vi "Sparameter Testing.vi"(0 "VNA Model:":enum16{"E5071C", "N5230A(C)", "N5224A"}(ring)=enum."N5224A", 1 "VNA VISA":refnum<visa-resource-name>="TCPIP0::A-N5224A-41544.local::hislip0::INSTR", 2 "Port Type":u16(ring), 3 "Reference":T2, 4 "VISA COM":refnum<visa-resource-name>="COM3", 5 "Channel":string="1", 6 "Information In":T1={"Sample PN: "="", "SampleSN:"="", "Sparam Test Item"=[], "S-para Pair Name"=[], "Length"="", "Diff Test Item Name"=["SDD21", "SDD22", "SCD21", "SCD22", "SCC11", "NEXT", "FEXT"], "Diff Test Item Name smooth"=[], "smooth point"=0.0, "limitSpec"=[], "switchIndexOffset"=0, "testType"=enum."Loss", "pairStartIndex"=0, "DAQ  Model:"=enum."NI PCI-6509", "VISA COM"="COM3", "Matrix  In"=[]}, 7 "TDR setting array":T3(array[cluster]), 8 "Mode(Demo,Manual)":T7, 9 "DAQ  Model:":T6(ring), 10 "S4P Data Type":enum16{"THRU", "NEXT", "FEXT"}(ring), 11 "Matrix  In":T8, 12 "ILDSpec":enum16{"IEEE802.3ba", "FDR", "EDR"}(ring), 13 "Option":T5, 14 "MulChannel?":bool, 15 "2X Thru":dbl[](array[numeric]), 16 "proBar_ref":refnum<vi>) -> (17 "String data":string, 18 "Basic Path":path, 19 "S4P_TXT_ Data":string[](array[string]), 20 "Frequency(Hz)":dbl[](array[numeric]), 21 "Data Out":dbl[][][](array[numeric]), 22 "Testing Results":bool[](array[boolean]), 24 "Total Reult":bool, 25 "TXT Data Path":path, 26 "Items Result":string[](array[string]), 27 "S4P Data Path":path)   [LabVIEW 2011]
uses:
  dataType/informationIn.ctl
  <userlib>/_OpenG.lib/array/array.llb/Delete Elements from 2D Array (DBL)__ogtk.vi
  <vilib>/Utility/file.llb/Write To Spreadsheet File (DBL).vi
  <vilib>/Utility/file.llb/Write To Spreadsheet File (string).vi
panel:
  in  "delay array":dbl[](array[numeric])
  out "Time Array 4":dbl[](array[numeric])
  out "Time Array 3":dbl[](array[numeric])
  out "NextSourced":dbl[][](array[numeric])
  in  "NEXT source":dbl[][](array[numeric])
  out "smoothed Diff Data":dbl[](array[numeric])
  out "ILD_15 graph index":i32
  out "reslut_TDD22toTDD11 2":bool
  out "reslut_TDD11toTDD22":bool
  out "1d reslut":bool[](array[boolean])
  out "TDD22toTDD11":dbl[](array[numeric])
  out "TDD11toTDD22":dbl[](array[numeric])
  out "Dataout":dbl[][](array[numeric])
  out "sparaLength":dbl
  in  "TDR Setting 2":T4
  out "Time Array 2":dbl[](array[numeric])
  out "SDD21 For ILD_15":dbl[][](array[numeric])
  out "大小":i32
  out "ILD_15%":bool[](array[boolean])
  out "ILD":dbl[][](array[numeric])
  out "Graph Size":i32
  in  "Skew result":dbl[](array[numeric])
  out "Skew Time":dbl[](array[numeric])=[4.0, 4.0015003751, 4.0030007502, 4.0045011253, 4.0060015004, 4.0075018755, 4.0090022506, 4.0105026257, 4.0120030008, 4.0135033758, 4.0150037509, 4.016504126, 4.0180045011, 4.0195048762, 4.0210052513, 4.0225056264, 4.0240060015, 4.0255063766, 4.0270067517, 4.0285071268, 4.0300075019, 4.031507877, 4.0330082521, 4.0345086272, 4.0360090023, 4.0375093773, 4.0390097524, 4.0405101275, 4.0420105026, 4.0435108777, 4.0450112528, 4.0465116279, 4.048012003, 4.0495123781, 4.0510127532, 4.0525131283, 4.0540135034, 4.0555138785, 4.0570142536, 4.0585146287, 4.0600150038, 4.0615153788, 4.0630157539, 4.064516129, 4.0660165041, 4.0675168792, 4.0690172543, 4.0705176294, 4.0720180045, 4.0735183796, 4.0750187547, 4.0765191298, 4.0780195049, 4.07951988, 4.0810202551, 4.0825206302, 4.0840210053, 4.0855213803, 4.0870217554, 4.0885221305, 4.0900225056, 4.0915228807, 4.0930232558, 4.0945236309, 4.096024006, 4.0975243811, 4.0990247562, 4.1005251313, 4.1020255064, 4.1035258815, 4.1050262566, 4.1065266317, 4.1080270068, 4.1095273818, 4.1110277569, 4.112528132, 4.1140285071, 4.1155288822, 4.1170292573, 4.1185296324, 4.1200300075, 4.1215303826, 4.1230307577, 4.1245311328, 4.1260315079, 4.127531883, 4.1290322581, 4.1305326332, 4.1320330083, 4.1335333833, 4.1350337584, 4.1365341335, 4.1380345086, 4.1395348837, 4.1410352588, 4.1425356339, 4.144036009, 4.1455363841, 4.1470367592, 4.1485371343, 4.1500375094, 4.1515378845, 4.1530382596, 4.1545386347, 4.1560390098, 4.1575393848, 4.1590397599, 4.160540135, 4.1620405101, 4.1635408852, 4.1650412603, 4.1665416354, 4.1680420105, 4.1695423856, 4.1710427607, 4.1725431358, 4.1740435109, 4.175543886, 4.1770442611, 4.1785446362, 4.1800450113, 4.1815453863, 4.1830457614, 4.1845461365, 4.1860465116, 4.1875468867, 4.1890472618, 4.1905476369, 4.192048012, 4.1935483871, 4.1950487622, 4.1965491373, 4.1980495124, 4.1995498875, 4.2010502626, 4.2025506377, 4.2040510128, 4.2055513878, 4.2070517629, 4.208552138, 4.2100525131, 4.2115528882, 4.2130532633, 4.2145536384, 4.2160540135, 4.2175543886, 4.2190547637, 4.2205551388, 4.2220555139, 4.223555889, 4.2250562641, 4.2265566392, 4.2280570143, 4.2295573893, 4.2310577644, 4.2325581395, 4.2340585146, 4.2355588897, 4.2370592648, 4.2385596399, 4.240060015, 4.2415603901, 4.2430607652, 4.2445611403, 4.2460615154, 4.2475618905, 4.2490622656, 4.2505626407, 4.2520630158, 4.2535633908, 4.2550637659, 4.256564141, 4.2580645161, 4.2595648912, 4.2610652663, 4.2625656414, 4.2640660165, 4.2655663916, 4.2670667667, 4.2685671418, 4.2700675169, 4.271567892, 4.2730682671, 4.2745686422, 4.2760690173, 4.2775693923, 4.2790697674, 4.2805701425, 4.2820705176, 4.2835708927, 4.2850712678, 4.2865716429, 4.288072018, 4.2895723931, 4.2910727682, 4.2925731433, 4.2940735184, 4.2955738935, 4.2970742686, 4.2985746437, 4.3000750188, 4.3015753938, 4.3030757689, 4.304576144, 4.3060765191, 4.3075768942, 4.3090772693, 4.3105776444, 4.3120780195, 4.3135783946, 4.3150787697, 4.3165791448, 4.3180795199, 4.319579895, 4.3210802701, 4.3225806452, 4.3240810203, 4.3255813953, 4.3270817704, 4.3285821455, 4.3300825206, 4.3315828957, 4.3330832708, 4.3345836459, 4.336084021, 4.3375843961, 4.3390847712, 4.3405851463, 4.3420855214, 4.3435858965, 4.3450862716, 4.3465866467, 4.3480870218, 4.3495873968, 4.3510877719, 4.352588147, 4.3540885221, 4.3555888972, 4.3570892723, 4.3585896474, 4.3600900225, 4.3615903976, 4.3630907727, 4.3645911478, 4.3660915229, 4.367591898, 4.3690922731, 4.3705926482, 4.3720930233, 4.3735933983, 4.3750937734, 4.3765941485, 4.3780945236, 4.3795948987, 4.3810952738, 4.3825956489, 4.384096024, 4.3855963991, 4.3870967742, 4.3885971493, 4.3900975244, 4.3915978995, 4.3930982746, 4.3945986497, 4.3960990248, 4.3975993998, 4.3990997749, 4.40060015, 4.4021005251, 4.4036009002, 4.4051012753, 4.4066016504, 4.4081020255, 4.4096024006, 4.4111027757, 4.4126031508, 4.4141035259, 4.415603901, 4.4171042761, 4.4186046512, 4.4201050263, 4.4216054014, 4.4231057764, 4.4246061515, 4.4261065266, 4.4276069017, 4.4291072768, 4.4306076519, 4.432108027, 4.4336084021, 4.4351087772, 4.4366091523, 4.4381095274, 4.4396099025, 4.4411102776, 4.4426106527, 4.4441110278, 4.4456114029, 4.4471117779, 4.448612153, 4.4501125281, 4.4516129032, 4.4531132783, 4.4546136534, 4.4561140285, 4.4576144036, 4.4591147787, 4.4606151538, 4.4621155289, 4.463615904, 4.4651162791, 4.4666166542, 4.4681170293, 4.4696174044, 4.4711177794, 4.4726181545, 4.4741185296, 4.4756189047, 4.4771192798, 4.4786196549, 4.48012003, 4.4816204051, 4.4831207802, 4.4846211553, 4.4861215304, 4.4876219055, 4.4891222806, 4.4906226557, 4.4921230308, 4.4936234059, 4.4951237809, 4.496624156, 4.4981245311, 4.4996249062, 4.5011252813, 4.5026256564, 4.5041260315, 4.5056264066, 4.5071267817, 4.5086271568, 4.5101275319, 4.511627907, 4.5131282821, 4.5146286572, 4.5161290323, 4.5176294074, 4.5191297824, 4.5206301575, 4.5221305326, 4.5236309077, 4.5251312828, 4.5266316579, 4.528132033, 4.5296324081, 4.5311327832, 4.5326331583, 4.5341335334, 4.5356339085, 4.5371342836, 4.5386346587, 4.5401350338, 4.5416354089, 4.5431357839, 4.544636159, 4.5461365341, 4.5476369092, 4.5491372843, 4.5506376594, 4.5521380345, 4.5536384096, 4.5551387847, 4.5566391598, 4.5581395349, 4.55963991, 4.5611402851, 4.5626406602, 4.5641410353, 4.5656414104, 4.5671417854, 4.5686421605, 4.5701425356, 4.5716429107, 4.5731432858, 4.5746436609, 4.576144036, 4.5776444111, 4.5791447862, 4.5806451613, 4.5821455364, 4.5836459115, 4.5851462866, 4.5866466617, 4.5881470368, 4.5896474119, 4.5911477869, 4.592648162, 4.5941485371, 4.5956489122, 4.5971492873, 4.5986496624, 4.6001500375, 4.6016504126, 4.6031507877, 4.6046511628, 4.6061515379, 4.607651913, 4.6091522881, 4.6106526632, 4.6121530383, 4.6136534134, 4.6151537884, 4.6166541635, 4.6181545386, 4.6196549137, 4.6211552888, 4.6226556639, 4.624156039, 4.6256564141, 4.6271567892, 4.6286571643, 4.6301575394, 4.6316579145, 4.6331582896, 4.6346586647, 4.6361590398, 4.6376594149, 4.6391597899, 4.640660165, 4.6421605401, 4.6436609152, 4.6451612903, 4.6466616654, 4.6481620405, 4.6496624156, 4.6511627907, 4.6526631658, 4.6541635409, 4.655663916, 4.6571642911, 4.6586646662, 4.6601650413, 4.6616654164, 4.6631657914, 4.6646661665, 4.6661665416, 4.6676669167, 4.6691672918, 4.6706676669, 4.672168042, 4.6736684171, 4.6751687922, 4.6766691673, 4.6781695424, 4.6796699175, 4.6811702926, 4.6826706677, 4.6841710428, 4.6856714179, 4.6871717929, 4.688672168, 4.6901725431, 4.6916729182, 4.6931732933, 4.6946736684, 4.6961740435, 4.6976744186, 4.6991747937, 4.7006751688, 4.7021755439, 4.703675919, 4.7051762941, 4.7066766692, 4.7081770443, 4.7096774194, 4.7111777944, 4.7126781695, 4.7141785446, 4.7156789197, 4.7171792948, 4.7186796699, 4.720180045, 4.7216804201, 4.7231807952, 4.7246811703, 4.7261815454, 4.7276819205, 4.7291822956, 4.7306826707, 4.7321830458, 4.7336834209, 4.7351837959, 4.736684171, 4.7381845461, 4.7396849212, 4.7411852963, 4.7426856714, 4.7441860465, 4.7456864216, 4.7471867967, 4.7486871718, 4.7501875469, 4.751687922, 4.7531882971, 4.7546886722, 4.7561890473, 4.7576894224, 4.7591897974, 4.7606901725, 4.7621905476, 4.7636909227, 4.7651912978, 4.7666916729, 4.768192048, 4.7696924231, 4.7711927982, 4.7726931733, 4.7741935484, 4.7756939235, 4.7771942986, 4.7786946737, 4.7801950488, 4.7816954239, 4.7831957989, 4.784696174, 4.7861965491, 4.7876969242, 4.7891972993, 4.7906976744, 4.7921980495, 4.7936984246, 4.7951987997, 4.7966991748, 4.7981995499, 4.799699925, 4.8012003001, 4.8027006752, 4.8042010503, 4.8057014254, 4.8072018005, 4.8087021755, 4.8102025506, 4.8117029257, 4.8132033008, 4.8147036759, 4.816204051, 4.8177044261, 4.8192048012, 4.8207051763, 4.8222055514, 4.8237059265, 4.8252063016, 4.8267066767, 4.8282070518, 4.8297074269, 4.831207802, 4.832708177, 4.8342085521, 4.8357089272, 4.8372093023, 4.8387096774, 4.8402100525, 4.8417104276, 4.8432108027, 4.8447111778, 4.8462115529, 4.847711928, 4.8492123031, 4.8507126782, 4.8522130533, 4.8537134284, 4.8552138035, 4.8567141785, 4.8582145536, 4.8597149287, 4.8612153038, 4.8627156789, 4.864216054, 4.8657164291, 4.8672168042, 4.8687171793, 4.8702175544, 4.8717179295, 4.8732183046, 4.8747186797, 4.8762190548, 4.8777194299, 4.879219805, 4.88072018, 4.8822205551, 4.8837209302, 4.8852213053, 4.8867216804, 4.8882220555, 4.8897224306, 4.8912228057, 4.8927231808, 4.8942235559, 4.895723931, 4.8972243061, 4.8987246812, 4.9002250563, 4.9017254314, 4.9032258065, 4.9047261815, 4.9062265566, 4.9077269317, 4.9092273068, 4.9107276819, 4.912228057, 4.9137284321, 4.9152288072, 4.9167291823, 4.9182295574, 4.9197299325, 4.9212303076, 4.9227306827, 4.9242310578, 4.9257314329, 4.927231808, 4.928732183, 4.9302325581, 4.9317329332, 4.9332333083, 4.9347336834, 4.9362340585, 4.9377344336, 4.9392348087, 4.9407351838, 4.9422355589, 4.943735934, 4.9452363091, 4.9467366842, 4.9482370593, 4.9497374344, 4.9512378095, 4.9527381845, 4.9542385596, 4.9557389347, 4.9572393098, 4.9587396849, 4.96024006, 4.9617404351, 4.9632408102, 4.9647411853, 4.9662415604, 4.9677419355, 4.9692423106, 4.9707426857, 4.9722430608, 4.9737434359, 4.975243811, 4.976744186, 4.9782445611, 4.9797449362, 4.9812453113, 4.9827456864, 4.9842460615, 4.9857464366, 4.9872468117, 4.9887471868, 4.9902475619, 4.991747937, 4.9932483121, 4.9947486872, 4.9962490623, 4.9977494374, 4.9992498125, 5.0007501875, 5.0022505626, 5.0037509377, 5.0052513128, 5.0067516879, 5.008252063, 5.0097524381, 5.0112528132, 5.0127531883, 5.0142535634, 5.0157539385, 5.0172543136, 5.0187546887, 5.0202550638, 5.0217554389, 5.023255814, 5.024756189, 5.0262565641, 5.0277569392, 5.0292573143, 5.0307576894, 5.0322580645, 5.0337584396, 5.0352588147, 5.0367591898, 5.0382595649, 5.03975994, 5.0412603151, 5.0427606902, 5.0442610653, 5.0457614404, 5.0472618155, 5.0487621905, 5.0502625656, 5.0517629407, 5.0532633158, 5.0547636909, 5.056264066, 5.0577644411, 5.0592648162, 5.0607651913, 5.0622655664, 5.0637659415, 5.0652663166, 5.0667666917, 5.0682670668, 5.0697674419, 5.071267817, 5.072768192, 5.0742685671, 5.0757689422, 5.0772693173, 5.0787696924, 5.0802700675, 5.0817704426, 5.0832708177, 5.0847711928, 5.0862715679, 5.087771943, 5.0892723181, 5.0907726932, 5.0922730683, 5.0937734434, 5.0952738185, 5.0967741935, 5.0982745686, 5.0997749437, 5.1012753188, 5.1027756939, 5.104276069, 5.1057764441, 5.1072768192, 5.1087771943, 5.1102775694, 5.1117779445, 5.1132783196, 5.1147786947, 5.1162790698, 5.1177794449, 5.11927982, 5.120780195, 5.1222805701, 5.1237809452, 5.1252813203, 5.1267816954, 5.1282820705, 5.1297824456, 5.1312828207, 5.1327831958, 5.1342835709, 5.135783946, 5.1372843211, 5.1387846962, 5.1402850713, 5.1417854464, 5.1432858215, 5.1447861965, 5.1462865716, 5.1477869467, 5.1492873218, 5.1507876969, 5.152288072, 5.1537884471, 5.1552888222, 5.1567891973, 5.1582895724, 5.1597899475, 5.1612903226, 5.1627906977, 5.1642910728, 5.1657914479, 5.167291823, 5.168792198, 5.1702925731, 5.1717929482, 5.1732933233, 5.1747936984, 5.1762940735, 5.1777944486, 5.1792948237, 5.1807951988, 5.1822955739, 5.183795949, 5.1852963241, 5.1867966992, 5.1882970743, 5.1897974494, 5.1912978245, 5.1927981995, 5.1942985746, 5.1957989497, 5.1972993248, 5.1987996999, 5.200300075, 5.2018004501, 5.2033008252, 5.2048012003, 5.2063015754, 5.2078019505, 5.2093023256, 5.2108027007, 5.2123030758, 5.2138034509, 5.215303826, 5.2168042011, 5.2183045761, 5.2198049512, 5.2213053263, 5.2228057014, 5.2243060765, 5.2258064516, 5.2273068267, 5.2288072018, 5.2303075769, 5.231807952, 5.2333083271, 5.2348087022, 5.2363090773, 5.2378094524, 5.2393098275, 5.2408102026, 5.2423105776, 5.2438109527, 5.2453113278, 5.2468117029, 5.248312078, 5.2498124531, 5.2513128282, 5.2528132033, 5.2543135784, 5.2558139535, 5.2573143286, 5.2588147037, 5.2603150788, 5.2618154539, 5.263315829, 5.2648162041, 5.2663165791, 5.2678169542, 5.2693173293, 5.2708177044, 5.2723180795, 5.2738184546, 5.2753188297, 5.2768192048, 5.2783195799, 5.279819955, 5.2813203301, 5.2828207052, 5.2843210803, 5.2858214554, 5.2873218305, 5.2888222056, 5.2903225806, 5.2918229557, 5.2933233308, 5.2948237059, 5.296324081, 5.2978244561, 5.2993248312, 5.3008252063, 5.3023255814, 5.3038259565, 5.3053263316, 5.3068267067, 5.3083270818, 5.3098274569, 5.311327832, 5.3128282071, 5.3143285821, 5.3158289572, 5.3173293323, 5.3188297074, 5.3203300825, 5.3218304576, 5.3233308327, 5.3248312078, 5.3263315829, 5.327831958, 5.3293323331, 5.3308327082, 5.3323330833, 5.3338334584, 5.3353338335, 5.3368342086, 5.3383345836, 5.3398349587, 5.3413353338, 5.3428357089, 5.344336084, 5.3458364591, 5.3473368342, 5.3488372093, 5.3503375844, 5.3518379595, 5.3533383346, 5.3548387097, 5.3563390848, 5.3578394599, 5.359339835, 5.3608402101, 5.3623405851, 5.3638409602, 5.3653413353, 5.3668417104, 5.3683420855, 5.3698424606, 5.3713428357, 5.3728432108, 5.3743435859, 5.375843961, 5.3773443361, 5.3788447112, 5.3803450863, 5.3818454614, 5.3833458365, 5.3848462116, 5.3863465866, 5.3878469617, 5.3893473368, 5.3908477119, 5.392348087, 5.3938484621, 5.3953488372, 5.3968492123, 5.3983495874, 5.3998499625, 5.4013503376, 5.4028507127, 5.4043510878, 5.4058514629, 5.407351838, 5.4088522131, 5.4103525881, 5.4118529632, 5.4133533383, 5.4148537134, 5.4163540885, 5.4178544636, 5.4193548387, 5.4208552138, 5.4223555889, 5.423855964, 5.4253563391, 5.4268567142, 5.4283570893, 5.4298574644, 5.4313578395, 5.4328582146, 5.4343585896, 5.4358589647, 5.4373593398, 5.4388597149, 5.44036009, 5.4418604651, 5.4433608402, 5.4448612153, 5.4463615904, 5.4478619655, 5.4493623406, 5.4508627157, 5.4523630908, 5.4538634659, 5.455363841, 5.4568642161, 5.4583645911, 5.4598649662, 5.4613653413, 5.4628657164, 5.4643660915, 5.4658664666, 5.4673668417, 5.4688672168, 5.4703675919, 5.471867967, 5.4733683421, 5.4748687172, 5.4763690923, 5.4778694674, 5.4793698425, 5.4808702176, 5.4823705926, 5.4838709677, 5.4853713428, 5.4868717179, 5.488372093, 5.4898724681, 5.4913728432, 5.4928732183, 5.4943735934, 5.4958739685, 5.4973743436, 5.4988747187, 5.5003750938, 5.5018754689, 5.503375844, 5.5048762191, 5.5063765941, 5.5078769692, 5.5093773443, 5.5108777194, 5.5123780945, 5.5138784696, 5.5153788447, 5.5168792198, 5.5183795949, 5.51987997, 5.5213803451, 5.5228807202, 5.5243810953, 5.5258814704, 5.5273818455, 5.5288822206, 5.5303825956, 5.5318829707, 5.5333833458, 5.5348837209, 5.536384096, 5.5378844711, 5.5393848462, 5.5408852213, 5.5423855964, 5.5438859715, 5.5453863466, 5.5468867217, 5.5483870968, 5.5498874719, 5.551387847, 5.5528882221, 5.5543885971, 5.5558889722, 5.5573893473, 5.5588897224, 5.5603900975, 5.5618904726, 5.5633908477, 5.5648912228, 5.5663915979, 5.567891973, 5.5693923481, 5.5708927232, 5.5723930983, 5.5738934734, 5.5753938485, 5.5768942236, 5.5783945986, 5.5798949737, 5.5813953488, 5.5828957239, 5.584396099, 5.5858964741, 5.5873968492, 5.5888972243, 5.5903975994, 5.5918979745, 5.5933983496, 5.5948987247, 5.5963990998, 5.5978994749, 5.59939985, 5.6009002251, 5.6024006002, 5.6039009752, 5.6054013503, 5.6069017254, 5.6084021005, 5.6099024756, 5.6114028507, 5.6129032258, 5.6144036009, 5.615903976, 5.6174043511, 5.6189047262, 5.6204051013, 5.6219054764, 5.6234058515, 5.6249062266, 5.6264066017, 5.6279069767, 5.6294073518, 5.6309077269, 5.632408102, 5.6339084771, 5.6354088522, 5.6369092273, 5.6384096024, 5.6399099775, 5.6414103526, 5.6429107277, 5.6444111028, 5.6459114779, 5.647411853, 5.6489122281, 5.6504126032, 5.6519129782, 5.6534133533, 5.6549137284, 5.6564141035, 5.6579144786, 5.6594148537, 5.6609152288, 5.6624156039, 5.663915979, 5.6654163541, 5.6669167292, 5.6684171043, 5.6699174794, 5.6714178545, 5.6729182296, 5.6744186047, 5.6759189797, 5.6774193548, 5.6789197299, 5.680420105, 5.6819204801, 5.6834208552, 5.6849212303, 5.6864216054, 5.6879219805, 5.6894223556, 5.6909227307, 5.6924231058, 5.6939234809, 5.695423856, 5.6969242311, 5.6984246062, 5.6999249812, 5.7014253563, 5.7029257314, 5.7044261065, 5.7059264816, 5.7074268567, 5.7089272318, 5.7104276069, 5.711927982, 5.7134283571, 5.7149287322, 5.7164291073, 5.7179294824, 5.7194298575, 5.7209302326, 5.7224306077, 5.7239309827, 5.7254313578, 5.7269317329, 5.728432108, 5.7299324831, 5.7314328582, 5.7329332333, 5.7344336084, 5.7359339835, 5.7374343586, 5.7389347337, 5.7404351088, 5.7419354839, 5.743435859, 5.7449362341, 5.7464366092, 5.7479369842, 5.7494373593, 5.7509377344, 5.7524381095, 5.7539384846, 5.7554388597, 5.7569392348, 5.7584396099, 5.759939985, 5.7614403601, 5.7629407352, 5.7644411103, 5.7659414854, 5.7674418605, 5.7689422356, 5.7704426107, 5.7719429857, 5.7734433608, 5.7749437359, 5.776444111, 5.7779444861, 5.7794448612, 5.7809452363, 5.7824456114, 5.7839459865, 5.7854463616, 5.7869467367, 5.7884471118, 5.7899474869, 5.791447862, 5.7929482371, 5.7944486122, 5.7959489872, 5.7974493623, 5.7989497374, 5.8004501125, 5.8019504876, 5.8034508627, 5.8049512378, 5.8064516129, 5.807951988, 5.8094523631, 5.8109527382, 5.8124531133, 5.8139534884, 5.8154538635, 5.8169542386, 5.8184546137, 5.8199549887, 5.8214553638, 5.8229557389, 5.824456114, 5.8259564891, 5.8274568642, 5.8289572393, 5.8304576144, 5.8319579895, 5.8334583646, 5.8349587397, 5.8364591148, 5.8379594899, 5.839459865, 5.8409602401, 5.8424606152, 5.8439609902, 5.8454613653, 5.8469617404, 5.8484621155, 5.8499624906, 5.8514628657, 5.8529632408, 5.8544636159, 5.855963991, 5.8574643661, 5.8589647412, 5.8604651163, 5.8619654914, 5.8634658665, 5.8649662416, 5.8664666167, 5.8679669917, 5.8694673668, 5.8709677419, 5.872468117, 5.8739684921, 5.8754688672, 5.8769692423, 5.8784696174, 5.8799699925, 5.8814703676, 5.8829707427, 5.8844711178, 5.8859714929, 5.887471868, 5.8889722431, 5.8904726182, 5.8919729932, 5.8934733683, 5.8949737434, 5.8964741185, 5.8979744936, 5.8994748687, 5.9009752438, 5.9024756189, 5.903975994, 5.9054763691, 5.9069767442, 5.9084771193, 5.9099774944, 5.9114778695, 5.9129782446, 5.9144786197, 5.9159789947, 5.9174793698, 5.9189797449, 5.92048012, 5.9219804951, 5.9234808702, 5.9249812453, 5.9264816204, 5.9279819955, 5.9294823706, 5.9309827457, 5.9324831208, 5.9339834959, 5.935483871, 5.9369842461, 5.9384846212, 5.9399849962, 5.9414853713, 5.9429857464, 5.9444861215, 5.9459864966, 5.9474868717, 5.9489872468, 5.9504876219, 5.951987997, 5.9534883721, 5.9549887472, 5.9564891223, 5.9579894974, 5.9594898725, 5.9609902476, 5.9624906227, 5.9639909977, 5.9654913728, 5.9669917479, 5.968492123, 5.9699924981, 5.9714928732, 5.9729932483, 5.9744936234, 5.9759939985, 5.9774943736, 5.9789947487, 5.9804951238, 5.9819954989, 5.983495874, 5.9849962491, 5.9864966242, 5.9879969992, 5.9894973743, 5.9909977494, 5.9924981245, 5.9939984996, 5.9954988747, 5.9969992498, 5.9984996249, 6.0, 6.0015003751, 6.0030007502, 6.0045011253, 6.0060015004, 6.0075018755, 6.0090022506, 6.0105026257, 6.0120030008, 6.0135033758, 6.0150037509, 6.016504126, 6.0180045011, 6.0195048762, 6.0210052513, 6.0225056264, 6.0240060015, 6.0255063766, 6.0270067517, 6.0285071268, 6.0300075019, 6.031507877, 6.0330082521, 6.0345086272, 6.0360090023, 6.0375093773, 6.0390097524, 6.0405101275, 6.0420105026, 6.0435108777, 6.0450112528, 6.0465116279, 6.048012003, 6.0495123781, 6.0510127532, 6.0525131283, 6.0540135034, 6.0555138785, 6.0570142536, 6.0585146287, 6.0600150038, 6.0615153788, 6.0630157539, 6.064516129, 6.0660165041, 6.0675168792, 6.0690172543, 6.0705176294, 6.0720180045, 6.0735183796, 6.0750187547, 6.0765191298, 6.0780195049, 6.07951988, 6.0810202551, 6.0825206302, 6.0840210053, 6.0855213803, 6.0870217554, 6.0885221305, 6.0900225056, 6.0915228807, 6.0930232558, 6.0945236309, 6.096024006, 6.0975243811, 6.0990247562, 6.1005251313, 6.1020255064, 6.1035258815, 6.1050262566, 6.1065266317, 6.1080270068, 6.1095273818, 6.1110277569, 6.112528132, 6.1140285071, 6.1155288822, 6.1170292573, 6.1185296324, 6.1200300075, 6.1215303826, 6.1230307577, 6.1245311328, 6.1260315079, 6.127531883, 6.1290322581, 6.1305326332, 6.1320330083, 6.1335333833, 6.1350337584, 6.1365341335, 6.1380345086, 6.1395348837, 6.1410352588, 6.1425356339, 6.144036009, 6.1455363841, 6.1470367592, 6.1485371343, 6.1500375094, 6.1515378845, 6.1530382596, 6.1545386347, 6.1560390098, 6.1575393848, 6.1590397599, 6.160540135, 6.1620405101, 6.1635408852, 6.1650412603, 6.1665416354, 6.1680420105, 6.1695423856, 6.1710427607, 6.1725431358, 6.1740435109, 6.175543886, 6.1770442611, 6.1785446362, 6.1800450113, 6.1815453863, 6.1830457614, 6.1845461365, 6.1860465116, 6.1875468867, 6.1890472618, 6.1905476369, 6.192048012, 6.1935483871, 6.1950487622, 6.1965491373, 6.1980495124, 6.1995498875, 6.2010502626, 6.2025506377, 6.2040510128, 6.2055513878, 6.2070517629, 6.208552138, 6.2100525131, 6.2115528882, 6.2130532633, 6.2145536384, 6.2160540135, 6.2175543886, 6.2190547637, 6.2205551388, 6.2220555139, 6.223555889, 6.2250562641, 6.2265566392, 6.2280570143, 6.2295573893, 6.2310577644, 6.2325581395, 6.2340585146, 6.2355588897, 6.2370592648, 6.2385596399, 6.240060015, 6.2415603901, 6.2430607652, 6.2445611403, 6.2460615154, 6.2475618905, 6.2490622656, 6.2505626407, 6.2520630158, 6.2535633908, 6.2550637659, 6.256564141, 6.2580645161, 6.2595648912, 6.2610652663, 6.2625656414, 6.2640660165, 6.2655663916, 6.2670667667, 6.2685671418, 6.2700675169, 6.271567892, 6.2730682671, 6.2745686422, 6.2760690173, 6.2775693923, 6.2790697674, 6.2805701425, 6.2820705176, 6.2835708927, 6.2850712678, 6.2865716429, 6.288072018, 6.2895723931, 6.2910727682, 6.2925731433, 6.2940735184, 6.2955738935, 6.2970742686, 6.2985746437, 6.3000750188, 6.3015753938, 6.3030757689, 6.304576144, 6.3060765191, 6.3075768942, 6.3090772693, 6.3105776444, 6.3120780195, 6.3135783946, 6.3150787697, 6.3165791448, 6.3180795199, 6.319579895, 6.3210802701, 6.3225806452, 6.3240810203, 6.3255813953, 6.3270817704, 6.3285821455, 6.3300825206, 6.3315828957, 6.3330832708, 6.3345836459, 6.336084021, 6.3375843961, 6.3390847712, 6.3405851463, 6.3420855214, 6.3435858965, 6.3450862716, 6.3465866467, 6.3480870218, 6.3495873968, 6.3510877719, 6.352588147, 6.3540885221, 6.3555888972, 6.3570892723, 6.3585896474, 6.3600900225, 6.3615903976, 6.3630907727, 6.3645911478, 6.3660915229, 6.367591898, 6.3690922731, 6.3705926482, 6.3720930233, 6.3735933983, 6.3750937734, 6.3765941485, 6.3780945236, 6.3795948987, 6.3810952738, 6.3825956489, 6.384096024, 6.3855963991, 6.3870967742, 6.3885971493, 6.3900975244, 6.3915978995, 6.3930982746, 6.3945986497, 6.3960990248, 6.3975993998, 6.3990997749, 6.40060015, 6.4021005251, 6.4036009002, 6.4051012753, 6.4066016504, 6.4081020255, 6.4096024006, 6.4111027757, 6.4126031508, 6.4141035259, 6.415603901, 6.4171042761, 6.4186046512, 6.4201050263, 6.4216054014, 6.4231057764, 6.4246061515, 6.4261065266, 6.4276069017, 6.4291072768, 6.4306076519, 6.432108027, 6.4336084021, 6.4351087772, 6.4366091523, 6.4381095274, 6.4396099025, 6.4411102776, 6.4426106527, 6.4441110278, 6.4456114029, 6.4471117779, 6.448612153, 6.4501125281, 6.4516129032, 6.4531132783, 6.4546136534, 6.4561140285, 6.4576144036, 6.4591147787, 6.4606151538, 6.4621155289, 6.463615904, 6.4651162791, 6.4666166542, 6.4681170293, 6.4696174044, 6.4711177794, 6.4726181545, 6.4741185296, 6.4756189047, 6.4771192798, 6.4786196549, 6.48012003, 6.4816204051, 6.4831207802, 6.4846211553, 6.4861215304, 6.4876219055, 6.4891222806, 6.4906226557, 6.4921230308, 6.4936234059, 6.4951237809, 6.496624156, 6.4981245311, 6.4996249062, 6.5011252813, 6.5026256564, 6.5041260315, 6.5056264066, 6.5071267817, 6.5086271568, 6.5101275319, 6.511627907, 6.5131282821, 6.5146286572, 6.5161290323, 6.5176294074, 6.5191297824, 6.5206301575, 6.5221305326, 6.5236309077, 6.5251312828, 6.5266316579, 6.528132033, 6.5296324081, 6.5311327832, 6.5326331583, 6.5341335334, 6.5356339085, 6.5371342836, 6.5386346587, 6.5401350338, 6.5416354089, 6.5431357839, 6.544636159, 6.5461365341, 6.5476369092, 6.5491372843, 6.5506376594, 6.5521380345, 6.5536384096, 6.5551387847, 6.5566391598, 6.5581395349, 6.55963991, 6.5611402851, 6.5626406602, 6.5641410353, 6.5656414104, 6.5671417854, 6.5686421605, 6.5701425356, 6.5716429107, 6.5731432858, 6.5746436609, 6.576144036, 6.5776444111, 6.5791447862, 6.5806451613, 6.5821455364, 6.5836459115, 6.5851462866, 6.5866466617, 6.5881470368, 6.5896474119, 6.5911477869, 6.592648162, 6.5941485371, 6.5956489122, 6.5971492873, 6.5986496624, 6.6001500375, 6.6016504126, 6.6031507877, 6.6046511628, 6.6061515379, 6.607651913, 6.6091522881, 6.6106526632, 6.6121530383, 6.6136534134, 6.6151537884, 6.6166541635, 6.6181545386, 6.6196549137, 6.6211552888, 6.6226556639, 6.624156039, 6.6256564141, 6.6271567892, 6.6286571643, 6.6301575394, 6.6316579145, 6.6331582896, 6.6346586647, 6.6361590398, 6.6376594149, 6.6391597899, 6.640660165, 6.6421605401, 6.6436609152, 6.6451612903, 6.6466616654, 6.6481620405, 6.6496624156, 6.6511627907, 6.6526631658, 6.6541635409, 6.655663916, 6.6571642911, 6.6586646662, 6.6601650413, 6.6616654164, 6.6631657914, 6.6646661665, 6.6661665416, 6.6676669167, 6.6691672918, 6.6706676669, 6.672168042, 6.6736684171, 6.6751687922, 6.6766691673, 6.6781695424, 6.6796699175, 6.6811702926, 6.6826706677, 6.6841710428, 6.6856714179, 6.6871717929, 6.688672168, 6.6901725431, 6.6916729182, 6.6931732933, 6.6946736684, 6.6961740435, 6.6976744186, 6.6991747937, 6.7006751688, 6.7021755439, 6.703675919, 6.7051762941, 6.7066766692, 6.7081770443, 6.7096774194, 6.7111777944, 6.7126781695, 6.7141785446, 6.7156789197, 6.7171792948, 6.7186796699, 6.720180045, 6.7216804201, 6.7231807952, 6.7246811703, 6.7261815454, 6.7276819205, 6.7291822956, 6.7306826707, 6.7321830458, 6.7336834209, 6.7351837959, 6.736684171, 6.7381845461, 6.7396849212, 6.7411852963, 6.7426856714, 6.7441860465, 6.7456864216, 6.7471867967, 6.7486871718, 6.7501875469, 6.751687922, 6.7531882971, 6.7546886722, 6.7561890473, 6.7576894224, 6.7591897974, 6.7606901725, 6.7621905476, 6.7636909227, 6.7651912978, 6.7666916729, 6.768192048, 6.7696924231, 6.7711927982, 6.7726931733, 6.7741935484, 6.7756939235, 6.7771942986, 6.7786946737, 6.7801950488, 6.7816954239, 6.7831957989, 6.784696174, 6.7861965491, 6.7876969242, 6.7891972993, 6.7906976744, 6.7921980495, 6.7936984246, 6.7951987997, 6.7966991748, 6.7981995499, 6.799699925, 6.8012003001, 6.8027006752, 6.8042010503, 6.8057014254, 6.8072018005, 6.8087021755, 6.8102025506, 6.8117029257, 6.8132033008, 6.8147036759, 6.816204051, 6.8177044261, 6.8192048012, 6.8207051763, 6.8222055514, 6.8237059265, 6.8252063016, 6.8267066767, 6.8282070518, 6.8297074269, 6.831207802, 6.832708177, 6.8342085521, 6.8357089272, 6.8372093023, 6.8387096774, 6.8402100525, 6.8417104276, 6.8432108027, 6.8447111778, 6.8462115529, 6.847711928, 6.8492123031, 6.8507126782, 6.8522130533, 6.8537134284, 6.8552138035, 6.8567141785, 6.8582145536, 6.8597149287, 6.8612153038, 6.8627156789, 6.864216054, 6.8657164291, 6.8672168042, 6.8687171793, 6.8702175544, 6.8717179295, 6.8732183046, 6.8747186797, 6.8762190548, 6.8777194299, 6.879219805, 6.88072018, 6.8822205551, 6.8837209302, 6.8852213053, 6.8867216804, 6.8882220555, 6.8897224306, 6.8912228057, 6.8927231808, 6.8942235559, 6.895723931, 6.8972243061, 6.8987246812, 6.9002250563, 6.9017254314, 6.9032258065, 6.9047261815, 6.9062265566, 6.9077269317, 6.9092273068, 6.9107276819, 6.912228057, 6.9137284321, 6.9152288072, 6.9167291823, 6.9182295574, 6.9197299325, 6.9212303076, 6.9227306827, 6.9242310578, 6.9257314329, 6.927231808, 6.928732183, 6.9302325581, 6.9317329332, 6.9332333083, 6.9347336834, 6.9362340585, 6.9377344336, 6.9392348087, 6.9407351838, 6.9422355589, 6.943735934, 6.9452363091, 6.9467366842, 6.9482370593, 6.9497374344, 6.9512378095, 6.9527381845, 6.9542385596, 6.9557389347, 6.9572393098, 6.9587396849, 6.96024006, 6.9617404351, 6.9632408102, 6.9647411853, 6.9662415604, 6.9677419355, 6.9692423106, 6.9707426857, 6.9722430608, 6.9737434359, 6.975243811, 6.976744186, 6.9782445611, 6.9797449362, 6.9812453113, 6.9827456864, 6.9842460615, 6.9857464366, 6.9872468117, 6.9887471868, 6.9902475619, 6.991747937, 6.9932483121, 6.9947486872, 6.9962490623, 6.9977494374, 6.9992498125, 7.0007501875, 7.0022505626, 7.0037509377, 7.0052513128, 7.0067516879, 7.008252063, 7.0097524381, 7.0112528132, 7.0127531883, 7.0142535634, 7.0157539385, 7.0172543136, 7.0187546887, 7.0202550638, 7.0217554389, 7.023255814, 7.024756189, 7.0262565641, 7.0277569392, 7.0292573143, 7.0307576894, 7.0322580645, 7.0337584396, 7.0352588147, 7.0367591898, 7.0382595649, 7.03975994, 7.0412603151, 7.0427606902, 7.0442610653, 7.0457614404, 7.0472618155, 7.0487621905, 7.0502625656, 7.0517629407, 7.0532633158, 7.0547636909, 7.056264066, 7.0577644411, 7.0592648162, 7.0607651913, 7.0622655664, 7.0637659415, 7.0652663166, 7.0667666917, 7.0682670668, 7.0697674419, 7.071267817, 7.072768192, 7.0742685671, 7.0757689422, 7.0772693173, 7.0787696924, 7.0802700675, 7.0817704426, 7.0832708177, 7.0847711928, 7.0862715679, 7.087771943, 7.0892723181, 7.0907726932, 7.0922730683, 7.0937734434, 7.0952738185, 7.0967741935, 7.0982745686, 7.0997749437, 7.1012753188, 7.1027756939, 7.104276069, 7.1057764441, 7.1072768192, 7.1087771943, 7.1102775694, 7.1117779445, 7.1132783196, 7.1147786947, 7.1162790698, 7.1177794449, 7.11927982, 7.120780195, 7.1222805701, 7.1237809452, 7.1252813203, 7.1267816954, 7.1282820705, 7.1297824456, 7.1312828207, 7.1327831958, 7.1342835709, 7.135783946, 7.1372843211, 7.1387846962, 7.1402850713, 7.1417854464, 7.1432858215, 7.1447861965, 7.1462865716, 7.1477869467, 7.1492873218, 7.1507876969, 7.152288072, 7.1537884471, 7.1552888222, 7.1567891973, 7.1582895724, 7.1597899475, 7.1612903226, 7.1627906977, 7.1642910728, 7.1657914479, 7.167291823, 7.168792198, 7.1702925731, 7.1717929482, 7.1732933233, 7.1747936984, 7.1762940735, 7.1777944486, 7.1792948237, 7.1807951988, 7.1822955739, 7.183795949, 7.1852963241, 7.1867966992, 7.1882970743, 7.1897974494, 7.1912978245, 7.1927981995, 7.1942985746, 7.1957989497, 7.1972993248, 7.1987996999, 7.200300075, 7.2018004501, 7.2033008252, 7.2048012003, 7.2063015754, 7.2078019505, 7.2093023256, 7.2108027007, 7.2123030758, 7.2138034509, 7.215303826, 7.2168042011, 7.2183045761, 7.2198049512, 7.2213053263, 7.2228057014, 7.2243060765, 7.2258064516, 7.2273068267, 7.2288072018, 7.2303075769, 7.231807952, 7.2333083271, 7.2348087022, 7.2363090773, 7.2378094524, 7.2393098275, 7.2408102026, 7.2423105776, 7.2438109527, 7.2453113278, 7.2468117029, 7.248312078, 7.2498124531, 7.2513128282, 7.2528132033, 7.2543135784, 7.2558139535, 7.2573143286, 7.2588147037, 7.2603150788, 7.2618154539, 7.263315829, 7.2648162041, 7.2663165791, 7.2678169542, 7.2693173293, 7.2708177044, 7.2723180795, 7.2738184546, 7.2753188297, 7.2768192048, 7.2783195799, 7.279819955, 7.2813203301, 7.2828207052, 7.2843210803, 7.2858214554, 7.2873218305, 7.2888222056, 7.2903225806, 7.2918229557, 7.2933233308, 7.2948237059, 7.296324081, 7.2978244561, 7.2993248312, 7.3008252063, 7.3023255814, 7.3038259565, 7.3053263316, 7.3068267067, 7.3083270818, 7.3098274569, 7.311327832, 7.3128282071, 7.3143285821, 7.3158289572, 7.3173293323, 7.3188297074, 7.3203300825, 7.3218304576, 7.3233308327, 7.3248312078, 7.3263315829, 7.327831958, 7.3293323331, 7.3308327082, 7.3323330833, 7.3338334584, 7.3353338335, 7.3368342086, 7.3383345836, 7.3398349587, 7.3413353338, 7.3428357089, 7.344336084, 7.3458364591, 7.3473368342, 7.3488372093, 7.3503375844, 7.3518379595, 7.3533383346, 7.3548387097, 7.3563390848, 7.3578394599, 7.359339835, 7.3608402101, 7.3623405851, 7.3638409602, 7.3653413353, 7.3668417104, 7.3683420855, 7.3698424606, 7.3713428357, 7.3728432108, 7.3743435859, 7.375843961, 7.3773443361, 7.3788447112, 7.3803450863, 7.3818454614, 7.3833458365, 7.3848462116, 7.3863465866, 7.3878469617, 7.3893473368, 7.3908477119, 7.392348087, 7.3938484621, 7.3953488372, 7.3968492123, 7.3983495874, 7.3998499625, 7.4013503376, 7.4028507127, 7.4043510878, 7.4058514629, 7.407351838, 7.4088522131, 7.4103525881, 7.4118529632, 7.4133533383, 7.4148537134, 7.4163540885, 7.4178544636, 7.4193548387, 7.4208552138, 7.4223555889, 7.423855964, 7.4253563391, 7.4268567142, 7.4283570893, 7.4298574644, 7.4313578395, 7.4328582146, 7.4343585896, 7.4358589647, 7.4373593398, 7.4388597149, 7.44036009, 7.4418604651, 7.4433608402, 7.4448612153, 7.4463615904, 7.4478619655, 7.4493623406, 7.4508627157, 7.4523630908, 7.4538634659, 7.455363841, 7.4568642161, 7.4583645911, 7.4598649662, 7.4613653413, 7.4628657164, 7.4643660915, 7.4658664666, 7.4673668417, 7.4688672168, 7.4703675919, 7.471867967, 7.4733683421, 7.4748687172, 7.4763690923, 7.4778694674, 7.4793698425, 7.4808702176, 7.4823705926, 7.4838709677, 7.4853713428, 7.4868717179, 7.488372093, 7.4898724681, 7.4913728432, 7.4928732183, 7.4943735934, 7.4958739685, 7.4973743436, 7.4988747187, 7.5003750938, 7.5018754689, 7.503375844, 7.5048762191, 7.5063765941, 7.5078769692, 7.5093773443, 7.5108777194, 7.5123780945, 7.5138784696, 7.5153788447, 7.5168792198, 7.5183795949, 7.51987997, 7.5213803451, 7.5228807202, 7.5243810953, 7.5258814704, 7.5273818455, 7.5288822206, 7.5303825956, 7.5318829707, 7.5333833458, 7.5348837209, 7.536384096, 7.5378844711, 7.5393848462, 7.5408852213, 7.5423855964, 7.5438859715, 7.5453863466, 7.5468867217, 7.5483870968, 7.5498874719, 7.551387847, 7.5528882221, 7.5543885971, 7.5558889722, 7.5573893473, 7.5588897224, 7.5603900975, 7.5618904726, 7.5633908477, 7.5648912228, 7.5663915979, 7.567891973, 7.5693923481, 7.5708927232, 7.5723930983, 7.5738934734, 7.5753938485, 7.5768942236, 7.5783945986, 7.5798949737, 7.5813953488, 7.5828957239, 7.584396099, 7.5858964741, 7.5873968492, 7.5888972243, 7.5903975994, 7.5918979745, 7.5933983496, 7.5948987247, 7.5963990998, 7.5978994749, 7.59939985, 7.6009002251, 7.6024006002, 7.6039009752, 7.6054013503, 7.6069017254, 7.6084021005, 7.6099024756, 7.6114028507, 7.6129032258, 7.6144036009, 7.615903976, 7.6174043511, 7.6189047262, 7.6204051013, 7.6219054764, 7.6234058515, 7.6249062266, 7.6264066017, 7.6279069767, 7.6294073518, 7.6309077269, 7.632408102, 7.6339084771, 7.6354088522, 7.6369092273, 7.6384096024, 7.6399099775, 7.6414103526, 7.6429107277, 7.6444111028, 7.6459114779, 7.647411853, 7.6489122281, 7.6504126032, 7.6519129782, 7.6534133533, 7.6549137284, 7.6564141035, 7.6579144786, 7.6594148537, 7.6609152288, 7.6624156039, 7.663915979, 7.6654163541, 7.6669167292, 7.6684171043, 7.6699174794, 7.6714178545, 7.6729182296, 7.6744186047, 7.6759189797, 7.6774193548, 7.6789197299, 7.680420105, 7.6819204801, 7.6834208552, 7.6849212303, 7.6864216054, 7.6879219805, 7.6894223556, 7.6909227307, 7.6924231058, 7.6939234809, 7.695423856, 7.6969242311, 7.6984246062, 7.6999249812, 7.7014253563, 7.7029257314, 7.7044261065, 7.7059264816, 7.7074268567, 7.7089272318, 7.7104276069, 7.711927982, 7.7134283571, 7.7149287322, 7.7164291073, 7.7179294824, 7.7194298575, 7.7209302326, 7.7224306077, 7.7239309827, 7.7254313578, 7.7269317329, 7.728432108, 7.7299324831, 7.7314328582, 7.7329332333, 7.7344336084, 7.7359339835, 7.7374343586, 7.7389347337, 7.7404351088, 7.7419354839, 7.743435859, 7.7449362341, 7.7464366092, 7.7479369842, 7.7494373593, 7.7509377344, 7.7524381095, 7.7539384846, 7.7554388597, 7.7569392348, 7.7584396099, 7.759939985, 7.7614403601, 7.7629407352, 7.7644411103, 7.7659414854, 7.7674418605, 7.7689422356, 7.7704426107, 7.7719429857, 7.7734433608, 7.7749437359, 7.776444111, 7.7779444861, 7.7794448612, 7.7809452363, 7.7824456114, 7.7839459865, 7.7854463616, 7.7869467367, 7.7884471118, 7.7899474869, 7.791447862, 7.7929482371, 7.7944486122, 7.7959489872, 7.7974493623, 7.7989497374, 7.8004501125, 7.8019504876, 7.8034508627, 7.8049512378, 7.8064516129, 7.807951988, 7.8094523631, 7.8109527382, 7.8124531133, 7.8139534884, 7.8154538635, 7.8169542386, 7.8184546137, 7.8199549887, 7.8214553638, 7.8229557389, 7.824456114, 7.8259564891, 7.8274568642, 7.8289572393, 7.8304576144, 7.8319579895, 7.8334583646, 7.8349587397, 7.8364591148, 7.8379594899, 7.839459865, 7.8409602401, 7.8424606152, 7.8439609902, 7.8454613653, 7.8469617404, 7.8484621155, 7.8499624906, 7.8514628657, 7.8529632408, 7.8544636159, 7.855963991, 7.8574643661, 7.8589647412, 7.8604651163, 7.8619654914, 7.8634658665, 7.8649662416, 7.8664666167, 7.8679669917, 7.8694673668, 7.8709677419, 7.872468117, 7.8739684921, 7.8754688672, 7.8769692423, 7.8784696174, 7.8799699925, 7.8814703676, 7.8829707427, 7.8844711178, 7.8859714929, 7.887471868, 7.8889722431, 7.8904726182, 7.8919729932, 7.8934733683, 7.8949737434, 7.8964741185, 7.8979744936, 7.8994748687, 7.9009752438, 7.9024756189, 7.903975994, 7.9054763691, 7.9069767442, 7.9084771193, 7.9099774944, 7.9114778695, 7.9129782446, 7.9144786197, 7.9159789947, 7.9174793698, 7.9189797449, 7.92048012, 7.9219804951, 7.9234808702, 7.9249812453, 7.9264816204, 7.9279819955, 7.9294823706, 7.9309827457, 7.9324831208, 7.9339834959, 7.935483871, 7.9369842461, 7.9384846212, 7.9399849962, 7.9414853713, 7.9429857464, 7.9444861215, 7.9459864966, 7.9474868717, 7.9489872468, 7.9504876219, 7.951987997, 7.9534883721, 7.9549887472, 7.9564891223, 7.9579894974, 7.9594898725, 7.9609902476, 7.9624906227, 7.9639909977, 7.9654913728, 7.9669917479, 7.968492123, 7.9699924981, 7.9714928732, 7.9729932483, 7.9744936234, 7.9759939985, 7.9774943736, 7.9789947487, 7.9804951238, 7.9819954989, 7.983495874, 7.9849962491, 7.9864966242, 7.9879969992, 7.9894973743, 7.9909977494, 7.9924981245, 7.9939984996, 7.9954988747, 7.9969992498, 7.9984996249, 8.0, 8.0015003751, 8.0030007502, 8.0045011253, 8.0060015004, 8.0075018755, 8.0090022506, 8.0105026257, 8.0120030008, 8.0135033758, 8.0150037509, 8.016504126, 8.0180045011, 8.0195048762, 8.0210052513, 8.0225056264, 8.0240060015, 8.0255063766, 8.0270067517, 8.0285071268, 8.0300075019, 8.031507877, 8.0330082521, 8.0345086272, 8.0360090023, 8.0375093773, 8.0390097524, 8.0405101275, 8.0420105026, 8.0435108777, 8.0450112528, 8.0465116279, 8.048012003, 8.0495123781, 8.0510127532, 8.0525131283, 8.0540135034, 8.0555138785, 8.0570142536, 8.0585146287, 8.0600150038, 8.0615153788, 8.0630157539, 8.064516129, 8.0660165041, 8.0675168792, 8.0690172543, 8.0705176294, 8.0720180045, 8.0735183796, 8.0750187547, 8.0765191298, 8.0780195049, 8.07951988, 8.0810202551, 8.0825206302, 8.0840210053, 8.0855213803, 8.0870217554, 8.0885221305, 8.0900225056, 8.0915228807, 8.0930232558, 8.0945236309, 8.096024006, 8.0975243811, 8.0990247562, 8.1005251313, 8.1020255064, 8.1035258815, 8.1050262566, 8.1065266317, 8.1080270068, 8.1095273818, 8.1110277569, 8.112528132, 8.1140285071, 8.1155288822, 8.1170292573, 8.1185296324, 8.1200300075, 8.1215303826, 8.1230307577, 8.1245311328, 8.1260315079, 8.127531883, 8.1290322581, 8.1305326332, 8.1320330083, 8.1335333833, 8.1350337584, 8.1365341335, 8.1380345086, 8.1395348837, 8.1410352588, 8.1425356339, 8.144036009, 8.1455363841, 8.1470367592, 8.1485371343, 8.1500375094, 8.1515378845, 8.1530382596, 8.1545386347, 8.1560390098, 8.1575393848, 8.1590397599, 8.160540135, 8.1620405101, 8.1635408852, 8.1650412603, 8.1665416354, 8.1680420105, 8.1695423856, 8.1710427607, 8.1725431358, 8.1740435109, 8.175543886, 8.1770442611, 8.1785446362, 8.1800450113, 8.1815453863, 8.1830457614, 8.1845461365, 8.1860465116, 8.1875468867, 8.1890472618, 8.1905476369, 8.192048012, 8.1935483871, 8.1950487622, 8.1965491373, 8.1980495124, 8.1995498875, 8.2010502626, 8.2025506377, 8.2040510128, 8.2055513878, 8.2070517629, 8.208552138, 8.2100525131, 8.2115528882, 8.2130532633, 8.2145536384, 8.2160540135, 8.2175543886, 8.2190547637, 8.2205551388, 8.2220555139, 8.223555889, 8.2250562641, 8.2265566392, 8.2280570143, 8.2295573893, 8.2310577644, 8.2325581395, 8.2340585146, 8.2355588897, 8.2370592648, 8.2385596399, 8.240060015, 8.2415603901, 8.2430607652, 8.2445611403, 8.2460615154, 8.2475618905, 8.2490622656, 8.2505626407, 8.2520630158, 8.2535633908, 8.2550637659, 8.256564141, 8.2580645161, 8.2595648912, 8.2610652663, 8.2625656414, 8.2640660165, 8.2655663916, 8.2670667667, 8.2685671418, 8.2700675169, 8.271567892, 8.2730682671, 8.2745686422, 8.2760690173, 8.2775693923, 8.2790697674, 8.2805701425, 8.2820705176, 8.2835708927, 8.2850712678, 8.2865716429, 8.288072018, 8.2895723931, 8.2910727682, 8.2925731433, 8.2940735184, 8.2955738935, 8.2970742686, 8.2985746437, 8.3000750188, 8.3015753938, 8.3030757689, 8.304576144, 8.3060765191, 8.3075768942, 8.3090772693, 8.3105776444, 8.3120780195, 8.3135783946, 8.3150787697, 8.3165791448, 8.3180795199, 8.319579895, 8.3210802701, 8.3225806452, 8.3240810203, 8.3255813953, 8.3270817704, 8.3285821455, 8.3300825206, 8.3315828957, 8.3330832708, 8.3345836459, 8.336084021, 8.3375843961, 8.3390847712, 8.3405851463, 8.3420855214, 8.3435858965, 8.3450862716, 8.3465866467, 8.3480870218, 8.3495873968, 8.3510877719, 8.352588147, 8.3540885221, 8.3555888972, 8.3570892723, 8.3585896474, 8.3600900225, 8.3615903976, 8.3630907727, 8.3645911478, 8.3660915229, 8.367591898, 8.3690922731, 8.3705926482, 8.3720930233, 8.3735933983, 8.3750937734, 8.3765941485, 8.3780945236, 8.3795948987, 8.3810952738, 8.3825956489, 8.384096024, 8.3855963991, 8.3870967742, 8.3885971493, 8.3900975244, 8.3915978995, 8.3930982746, 8.3945986497, 8.3960990248, 8.3975993998, 8.3990997749, 8.40060015, 8.4021005251, 8.4036009002, 8.4051012753, 8.4066016504, 8.4081020255, 8.4096024006, 8.4111027757, 8.4126031508, 8.4141035259, 8.415603901, 8.4171042761, 8.4186046512, 8.4201050263, 8.4216054014, 8.4231057764, 8.4246061515, 8.4261065266, 8.4276069017, 8.4291072768, 8.4306076519, 8.432108027, 8.4336084021, 8.4351087772, 8.4366091523, 8.4381095274, 8.4396099025, 8.4411102776, 8.4426106527, 8.4441110278, 8.4456114029, 8.4471117779, 8.448612153, 8.4501125281, 8.4516129032, 8.4531132783, 8.4546136534, 8.4561140285, 8.4576144036, 8.4591147787, 8.4606151538, 8.4621155289, 8.463615904, 8.4651162791, 8.4666166542, 8.4681170293, 8.4696174044, 8.4711177794, 8.4726181545, 8.4741185296, 8.4756189047, 8.4771192798, 8.4786196549, 8.48012003, 8.4816204051, 8.4831207802, 8.4846211553, 8.4861215304, 8.4876219055, 8.4891222806, 8.4906226557, 8.4921230308, 8.4936234059, 8.4951237809, 8.496624156, 8.4981245311, 8.4996249062, 8.5011252813, 8.5026256564, 8.5041260315, 8.5056264066, 8.5071267817, 8.5086271568, 8.5101275319, 8.511627907, 8.5131282821, 8.5146286572, 8.5161290323, 8.5176294074, 8.5191297824, 8.5206301575, 8.5221305326, 8.5236309077, 8.5251312828, 8.5266316579, 8.528132033, 8.5296324081, 8.5311327832, 8.5326331583, 8.5341335334, 8.5356339085, 8.5371342836, 8.5386346587, 8.5401350338, 8.5416354089, 8.5431357839, 8.544636159, 8.5461365341, 8.5476369092, 8.5491372843, 8.5506376594, 8.5521380345, 8.5536384096, 8.5551387847, 8.5566391598, 8.5581395349, 8.55963991, 8.5611402851, 8.5626406602, 8.5641410353, 8.5656414104, 8.5671417854, 8.5686421605, 8.5701425356, 8.5716429107, 8.5731432858, 8.5746436609, 8.576144036, 8.5776444111, 8.5791447862, 8.5806451613, 8.5821455364, 8.5836459115, 8.5851462866, 8.5866466617, 8.5881470368, 8.5896474119, 8.5911477869, 8.592648162, 8.5941485371, 8.5956489122, 8.5971492873, 8.5986496624, 8.6001500375, 8.6016504126, 8.6031507877, 8.6046511628, 8.6061515379, 8.607651913, 8.6091522881, 8.6106526632, 8.6121530383, 8.6136534134, 8.6151537884, 8.6166541635, 8.6181545386, 8.6196549137, 8.6211552888, 8.6226556639, 8.624156039, 8.6256564141, 8.6271567892, 8.6286571643, 8.6301575394, 8.6316579145, 8.6331582896, 8.6346586647, 8.6361590398, 8.6376594149, 8.6391597899, 8.640660165, 8.6421605401, 8.6436609152, 8.6451612903, 8.6466616654, 8.6481620405, 8.6496624156, 8.6511627907, 8.6526631658, 8.6541635409, 8.655663916, 8.6571642911, 8.6586646662, 8.6601650413, 8.6616654164, 8.6631657914, 8.6646661665, 8.6661665416, 8.6676669167, 8.6691672918, 8.6706676669, 8.672168042, 8.6736684171, 8.6751687922, 8.6766691673, 8.6781695424, 8.6796699175, 8.6811702926, 8.6826706677, 8.6841710428, 8.6856714179, 8.6871717929, 8.688672168, 8.6901725431, 8.6916729182, 8.6931732933, 8.6946736684, 8.6961740435, 8.6976744186, 8.6991747937, 8.7006751688, 8.7021755439, 8.703675919, 8.7051762941, 8.7066766692, 8.7081770443, 8.7096774194, 8.7111777944, 8.7126781695, 8.7141785446, 8.7156789197, 8.7171792948, 8.7186796699, 8.720180045, 8.7216804201, 8.7231807952, 8.7246811703, 8.7261815454, 8.7276819205, 8.7291822956, 8.7306826707, 8.7321830458, 8.7336834209, 8.7351837959, 8.736684171, 8.7381845461, 8.7396849212, 8.7411852963, 8.7426856714, 8.7441860465, 8.7456864216, 8.7471867967, 8.7486871718, 8.7501875469, 8.751687922, 8.7531882971, 8.7546886722, 8.7561890473, 8.7576894224, 8.7591897974, 8.7606901725, 8.7621905476, 8.7636909227, 8.7651912978, 8.7666916729, 8.768192048, 8.7696924231, 8.7711927982, 8.7726931733, 8.7741935484, 8.7756939235, 8.7771942986, 8.7786946737, 8.7801950488, 8.7816954239, 8.7831957989, 8.784696174, 8.7861965491, 8.7876969242, 8.7891972993, 8.7906976744, 8.7921980495, 8.7936984246, 8.7951987997, 8.7966991748, 8.7981995499, 8.799699925, 8.8012003001, 8.8027006752, 8.8042010503, 8.8057014254, 8.8072018005, 8.8087021755, 8.8102025506, 8.8117029257, 8.8132033008, 8.8147036759, 8.816204051, 8.8177044261, 8.8192048012, 8.8207051763, 8.8222055514, 8.8237059265, 8.8252063016, 8.8267066767, 8.8282070518, 8.8297074269, 8.831207802, 8.832708177, 8.8342085521, 8.8357089272, 8.8372093023, 8.8387096774, 8.8402100525, 8.8417104276, 8.8432108027, 8.8447111778, 8.8462115529, 8.847711928, 8.8492123031, 8.8507126782, 8.8522130533, 8.8537134284, 8.8552138035, 8.8567141785, 8.8582145536, 8.8597149287, 8.8612153038, 8.8627156789, 8.864216054, 8.8657164291, 8.8672168042, 8.8687171793, 8.8702175544, 8.8717179295, 8.8732183046, 8.8747186797, 8.8762190548, 8.8777194299, 8.879219805, 8.88072018, 8.8822205551, 8.8837209302, 8.8852213053, 8.8867216804, 8.8882220555, 8.8897224306, 8.8912228057, 8.8927231808, 8.8942235559, 8.895723931, 8.8972243061, 8.8987246812, 8.9002250563, 8.9017254314, 8.9032258065, 8.9047261815, 8.9062265566, 8.9077269317, 8.9092273068, 8.9107276819, 8.912228057, 8.9137284321, 8.9152288072, 8.9167291823, 8.9182295574, 8.9197299325, 8.9212303076, 8.9227306827, 8.9242310578, 8.9257314329, 8.927231808, 8.928732183, 8.9302325581, 8.9317329332, 8.9332333083, 8.9347336834, 8.9362340585, 8.9377344336, 8.9392348087, 8.9407351838, 8.9422355589, 8.943735934, 8.9452363091, 8.9467366842, 8.9482370593, 8.9497374344, 8.9512378095, 8.9527381845, 8.9542385596, 8.9557389347, 8.9572393098, 8.9587396849, 8.96024006, 8.9617404351, 8.9632408102, 8.9647411853, 8.9662415604, 8.9677419355, 8.9692423106, 8.9707426857, 8.9722430608, 8.9737434359, 8.975243811, 8.976744186, 8.9782445611, 8.9797449362, 8.9812453113, 8.9827456864, 8.9842460615, 8.9857464366, 8.9872468117, 8.9887471868, 8.9902475619, 8.991747937, 8.9932483121, 8.9947486872, 8.9962490623, 8.9977494374, 8.9992498125, 9.0007501875, 9.0022505626, 9.0037509377, 9.0052513128, 9.0067516879, 9.008252063, 9.0097524381, 9.0112528132, 9.0127531883, 9.0142535634, 9.0157539385, 9.0172543136, 9.0187546887, 9.0202550638, 9.0217554389, 9.023255814, 9.024756189, 9.0262565641, 9.0277569392, 9.0292573143, 9.0307576894, 9.0322580645, 9.0337584396, 9.0352588147, 9.0367591898, 9.0382595649, 9.03975994, 9.0412603151, 9.0427606902, 9.0442610653, 9.0457614404, 9.0472618155, 9.0487621905, 9.0502625656, 9.0517629407, 9.0532633158, 9.0547636909, 9.056264066, 9.0577644411, 9.0592648162, 9.0607651913, 9.0622655664, 9.0637659415, 9.0652663166, 9.0667666917, 9.0682670668, 9.0697674419, 9.071267817, 9.072768192, 9.0742685671, 9.0757689422, 9.0772693173, 9.0787696924, 9.0802700675, 9.0817704426, 9.0832708177, 9.0847711928, 9.0862715679, 9.087771943, 9.0892723181, 9.0907726932, 9.0922730683, 9.0937734434, 9.0952738185, 9.0967741935, 9.0982745686, 9.0997749437, 9.1012753188, 9.1027756939, 9.104276069, 9.1057764441, 9.1072768192, 9.1087771943, 9.1102775694, 9.1117779445, 9.1132783196, 9.1147786947, 9.1162790698, 9.1177794449, 9.11927982, 9.120780195, 9.1222805701, 9.1237809452, 9.1252813203, 9.1267816954, 9.1282820705, 9.1297824456, 9.1312828207, 9.1327831958, 9.1342835709, 9.135783946, 9.1372843211, 9.1387846962, 9.1402850713, 9.1417854464, 9.1432858215, 9.1447861965, 9.1462865716, 9.1477869467, 9.1492873218, 9.1507876969, 9.152288072, 9.1537884471, 9.1552888222, 9.1567891973, 9.1582895724, 9.1597899475, 9.1612903226, 9.1627906977, 9.1642910728, 9.1657914479, 9.167291823, 9.168792198, 9.1702925731, 9.1717929482, 9.1732933233, 9.1747936984, 9.1762940735, 9.1777944486, 9.1792948237, 9.1807951988, 9.1822955739, 9.183795949, 9.1852963241, 9.1867966992, 9.1882970743, 9.1897974494, 9.1912978245, 9.1927981995, 9.1942985746, 9.1957989497, 9.1972993248, 9.1987996999, 9.200300075, 9.2018004501, 9.2033008252, 9.2048012003, 9.2063015754, 9.2078019505, 9.2093023256, 9.2108027007, 9.2123030758, 9.2138034509, 9.215303826, 9.2168042011, 9.2183045761, 9.2198049512, 9.2213053263, 9.2228057014, 9.2243060765, 9.2258064516, 9.2273068267, 9.2288072018, 9.2303075769, 9.231807952, 9.2333083271, 9.2348087022, 9.2363090773, 9.2378094524, 9.2393098275, 9.2408102026, 9.2423105776, 9.2438109527, 9.2453113278, 9.2468117029, 9.248312078, 9.2498124531, 9.2513128282, 9.2528132033, 9.2543135784, 9.2558139535, 9.2573143286, 9.2588147037, 9.2603150788, 9.2618154539, 9.263315829, 9.2648162041, 9.2663165791, 9.2678169542, 9.2693173293, 9.2708177044, 9.2723180795, 9.2738184546, 9.2753188297, 9.2768192048, 9.2783195799, 9.279819955, 9.2813203301, 9.2828207052, 9.2843210803, 9.2858214554, 9.2873218305, 9.2888222056, 9.2903225806, 9.2918229557, 9.2933233308, 9.2948237059, 9.296324081, 9.2978244561, 9.2993248312, 9.3008252063, 9.3023255814, 9.3038259565, 9.3053263316, 9.3068267067, 9.3083270818, 9.3098274569, 9.311327832, 9.3128282071, 9.3143285821, 9.3158289572, 9.3173293323, 9.3188297074, 9.3203300825, 9.3218304576, 9.3233308327, 9.3248312078, 9.3263315829, 9.327831958, 9.3293323331, 9.3308327082, 9.3323330833, 9.3338334584, 9.3353338335, 9.3368342086, 9.3383345836, 9.3398349587, 9.3413353338, 9.3428357089, 9.344336084, 9.3458364591, 9.3473368342, 9.3488372093, 9.3503375844, 9.3518379595, 9.3533383346, 9.3548387097, 9.3563390848, 9.3578394599, 9.359339835, 9.3608402101, 9.3623405851, 9.3638409602, 9.3653413353, 9.3668417104, 9.3683420855, 9.3698424606, 9.3713428357, 9.3728432108, 9.3743435859, 9.375843961, 9.3773443361, 9.3788447112, 9.3803450863, 9.3818454614, 9.3833458365, 9.3848462116, 9.3863465866, 9.3878469617, 9.3893473368, 9.3908477119, 9.392348087, 9.3938484621, 9.3953488372, 9.3968492123, 9.3983495874, 9.3998499625, 9.4013503376, 9.4028507127, 9.4043510878, 9.4058514629, 9.407351838, 9.4088522131, 9.4103525881, 9.4118529632, 9.4133533383, 9.4148537134, 9.4163540885, 9.4178544636, 9.4193548387, 9.4208552138, 9.4223555889, 9.423855964, 9.4253563391, 9.4268567142, 9.4283570893, 9.4298574644, 9.4313578395, 9.4328582146, 9.4343585896, 9.4358589647, 9.4373593398, 9.4388597149, 9.44036009, 9.4418604651, 9.4433608402, 9.4448612153, 9.4463615904, 9.4478619655, 9.4493623406, 9.4508627157, 9.4523630908, 9.4538634659, 9.455363841, 9.4568642161, 9.4583645911, 9.4598649662, 9.4613653413, 9.4628657164, 9.4643660915, 9.4658664666, 9.4673668417, 9.4688672168, 9.4703675919, 9.471867967, 9.4733683421, 9.4748687172, 9.4763690923, 9.4778694674, 9.4793698425, 9.4808702176, 9.4823705926, 9.4838709677, 9.4853713428, 9.4868717179, 9.488372093, 9.4898724681, 9.4913728432, 9.4928732183, 9.4943735934, 9.4958739685, 9.4973743436, 9.4988747187, 9.5003750938, 9.5018754689, 9.503375844, 9.5048762191, 9.5063765941, 9.5078769692, 9.5093773443, 9.5108777194, 9.5123780945, 9.5138784696, 9.5153788447, 9.5168792198, 9.5183795949, 9.51987997, 9.5213803451, 9.5228807202, 9.5243810953, 9.5258814704, 9.5273818455, 9.5288822206, 9.5303825956, 9.5318829707, 9.5333833458, 9.5348837209, 9.536384096, 9.5378844711, 9.5393848462, 9.5408852213, 9.5423855964, 9.5438859715, 9.5453863466, 9.5468867217, 9.5483870968, 9.5498874719, 9.551387847, 9.5528882221, 9.5543885971, 9.5558889722, 9.5573893473, 9.5588897224, 9.5603900975, 9.5618904726, 9.5633908477, 9.5648912228, 9.5663915979, 9.567891973, 9.5693923481, 9.5708927232, 9.5723930983, 9.5738934734, 9.5753938485, 9.5768942236, 9.5783945986, 9.5798949737, 9.5813953488, 9.5828957239, 9.584396099, 9.5858964741, 9.5873968492, 9.5888972243, 9.5903975994, 9.5918979745, 9.5933983496, 9.5948987247, 9.5963990998, 9.5978994749, 9.59939985, 9.6009002251, 9.6024006002, 9.6039009752, 9.6054013503, 9.6069017254, 9.6084021005, 9.6099024756, 9.6114028507, 9.6129032258, 9.6144036009, 9.615903976, 9.6174043511, 9.6189047262, 9.6204051013, 9.6219054764, 9.6234058515, 9.6249062266, 9.6264066017, 9.6279069767, 9.6294073518, 9.6309077269, 9.632408102, 9.6339084771, 9.6354088522, 9.6369092273, 9.6384096024, 9.6399099775, 9.6414103526, 9.6429107277, 9.6444111028, 9.6459114779, 9.647411853, 9.6489122281, 9.6504126032, 9.6519129782, 9.6534133533, 9.6549137284, 9.6564141035, 9.6579144786, 9.6594148537, 9.6609152288, 9.6624156039, 9.663915979, 9.6654163541, 9.6669167292, 9.6684171043, 9.6699174794, 9.6714178545, 9.6729182296, 9.6744186047, 9.6759189797, 9.6774193548, 9.6789197299, 9.680420105, 9.6819204801, 9.6834208552, 9.6849212303, 9.6864216054, 9.6879219805, 9.6894223556, 9.6909227307, 9.6924231058, 9.6939234809, 9.695423856, 9.6969242311, 9.6984246062, 9.6999249812, 9.7014253563, 9.7029257314, 9.7044261065, 9.7059264816, 9.7074268567, 9.7089272318, 9.7104276069, 9.711927982, 9.7134283571, 9.7149287322, 9.7164291073, 9.7179294824, 9.7194298575, 9.7209302326, 9.7224306077, 9.7239309827, 9.7254313578, 9.7269317329, 9.728432108, 9.7299324831, 9.7314328582, 9.7329332333, 9.7344336084, 9.7359339835, 9.7374343586, 9.7389347337, 9.7404351088, 9.7419354839, 9.743435859, 9.7449362341, 9.7464366092, 9.7479369842, 9.7494373593, 9.7509377344, 9.7524381095, 9.7539384846, 9.7554388597, 9.7569392348, 9.7584396099, 9.759939985, 9.7614403601, 9.7629407352, 9.7644411103, 9.7659414854, 9.7674418605, 9.7689422356, 9.7704426107, 9.7719429857, 9.7734433608, 9.7749437359, 9.776444111, 9.7779444861, 9.7794448612, 9.7809452363, 9.7824456114, 9.7839459865, 9.7854463616, 9.7869467367, 9.7884471118, 9.7899474869, 9.791447862, 9.7929482371, 9.7944486122, 9.7959489872, 9.7974493623, 9.7989497374, 9.8004501125, 9.8019504876, 9.8034508627, 9.8049512378, 9.8064516129, 9.807951988, 9.8094523631, 9.8109527382, 9.8124531133, 9.8139534884, 9.8154538635, 9.8169542386, 9.8184546137, 9.8199549887, 9.8214553638, 9.8229557389, 9.824456114, 9.8259564891, 9.8274568642, 9.8289572393, 9.8304576144, 9.8319579895, 9.8334583646, 9.8349587397, 9.8364591148, 9.8379594899, 9.839459865, 9.8409602401, 9.8424606152, 9.8439609902, 9.8454613653, 9.8469617404, 9.8484621155, 9.8499624906, 9.8514628657, 9.8529632408, 9.8544636159, 9.855963991, 9.8574643661, 9.8589647412, 9.8604651163, 9.8619654914, 9.8634658665, 9.8649662416, 9.8664666167, 9.8679669917, 9.8694673668, 9.8709677419, 9.872468117, 9.8739684921, 9.8754688672, 9.8769692423, 9.8784696174, 9.8799699925, 9.8814703676, 9.8829707427, 9.8844711178, 9.8859714929, 9.887471868, 9.8889722431, 9.8904726182, 9.8919729932, 9.8934733683, 9.8949737434, 9.8964741185, 9.8979744936, 9.8994748687, 9.9009752438, 9.9024756189, 9.903975994, 9.9054763691, 9.9069767442, 9.9084771193, 9.9099774944, 9.9114778695, 9.9129782446, 9.9144786197, 9.9159789947, 9.9174793698, 9.9189797449, 9.92048012, 9.9219804951, 9.9234808702, 9.9249812453, 9.9264816204, 9.9279819955, 9.9294823706, 9.9309827457, 9.9324831208, 9.9339834959, 9.935483871, 9.9369842461, 9.9384846212, 9.9399849962, 9.9414853713, 9.9429857464, 9.9444861215, 9.9459864966, 9.9474868717, 9.9489872468, 9.9504876219, 9.951987997, 9.9534883721, 9.9549887472, 9.9564891223, 9.9579894974, 9.9594898725, 9.9609902476, 9.9624906227, 9.9639909977, 9.9654913728, 9.9669917479, 9.968492123, 9.9699924981, 9.9714928732, 9.9729932483, 9.9744936234, 9.9759939985, 9.9774943736, 9.9789947487, 9.9804951238, 9.9819954989, 9.983495874, 9.9849962491, 9.9864966242, 9.9879969992, 9.9894973743, 9.9909977494, 9.9924981245, 9.9939984996, 9.9954988747, 9.9969992498, 9.9984996249, 10.0]
  out "Size":i32
  out "Time Array":dbl[](array[numeric])
  out "S4P File Path":path
  out "Result":bool[][](array[boolean])
  out "Single  Data":dbl[][](array[numeric])
  out "Diff Data":dbl[][](array[numeric])
  in  "S4P Fomat":enum16{"RI", "dB"}(ring)
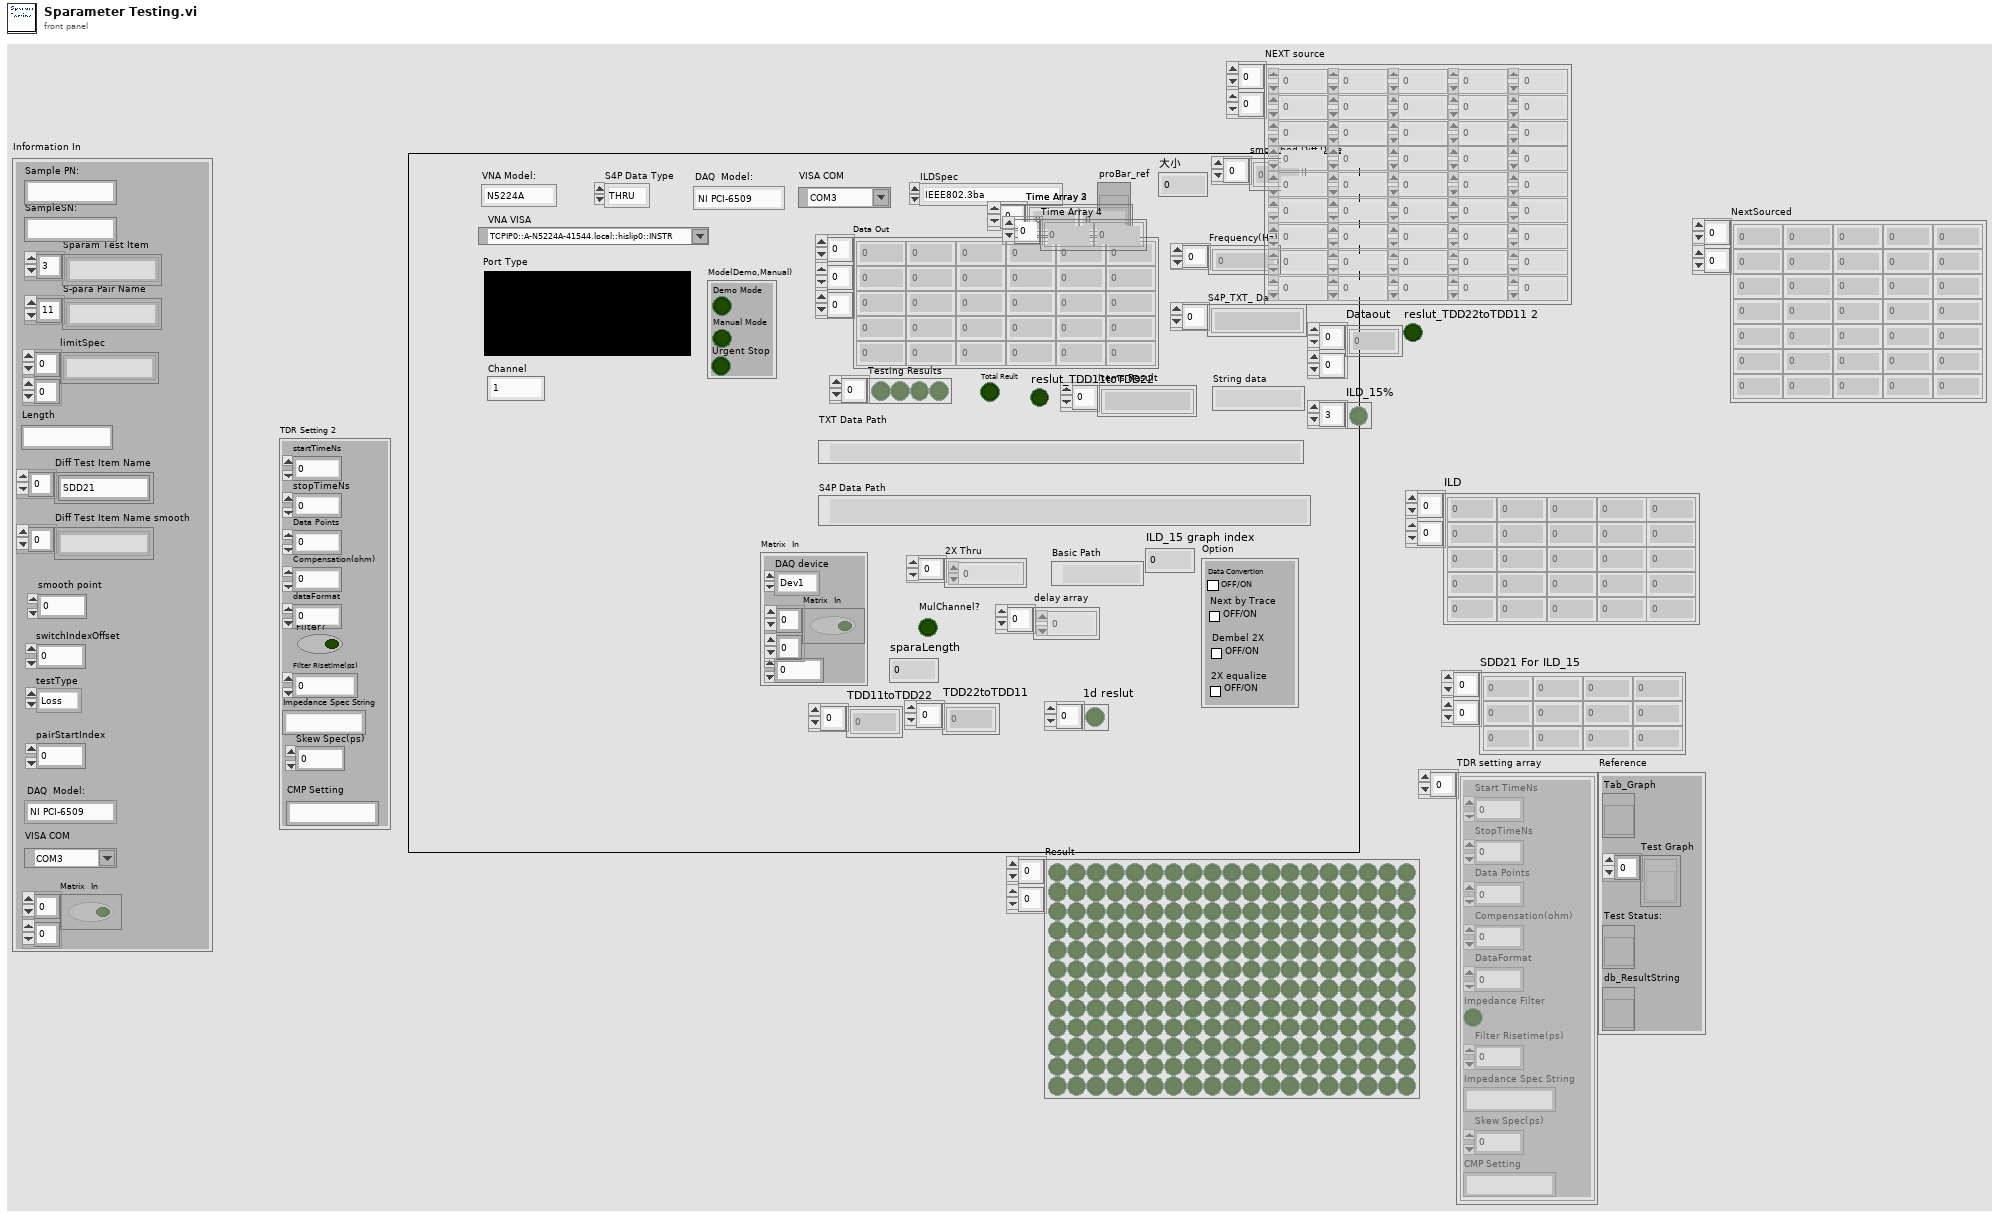
[diagram p1: front panel]
types:
  T1 = typedef "informationIn.ctl" = cluster{"Sample PN: ":string, "SampleSN:":string, "Sparam Test Item":string[], "S-para Pair Name":string[], "Length":string, "Diff Test Item Name":string[], "Diff Test Item Name smooth":string[], "smooth point":dbl, "limitSpec":string[][], "switchIndexOffset":i32, "testType":enum16{"Loss", "Next", "Fext"}, "pairStartIndex":i32, "DAQ  Model:":enum16{"NI PCI-6509", "LX MCU", "LX MCU_40G", "LX MCU_40G_HuaWei"}, "VISA COM":refnum<visa-resource-name>, "Matrix  In":bool[][]}
  T2 = cluster{"Tab_Graph":refnum<vi>, "Test Graph":refnum<vi>[], "Test Status:":refnum<vi>, "db_ResultString":refnum<vi>}
  T3 = cluster{"Start TimeNs":dbl, "StopTimeNs":dbl, "Data Points":i32, "Compensation(ohm)":dbl, "DataFormat":i16, "Impedance Filter":bool, "Filter Risetime(ps)":dbl, "Impedance Spec String":string, "Skew Spec(ps)":i32, "CMP Setting":string}[]
  T4 = cluster{"startTimeNs":dbl, "stopTimeNs":dbl, "Data Points":i32, "Compensation(ohm)":dbl, "dataFormat":i16, "Filter?":bool, "Filter Risetime(ps)":dbl, "Impedance Spec String":string, "Skew Spec(ps)":i32, "CMP Setting":string}
  T5 = cluster{"Data Convertion":bool, "Next by Trace":bool, "Dembel 2X":bool, "2X equalize ":bool}
  T6 = enum16{"NI PCI-6509", "LX MCU", "LX MCU_40G", "LX MCU_40G_HuaWei"}
  T7 = cluster{"Demo Mode":bool, "Manual Mode":bool, "Urgent Stop":bool}
  T8 = cluster{"DAQ device":enum16{"Dev1", "Dev2", "Dev3"}, "Matrix  In":bool[][], i32}
  T9 = cluster{"Start TimeNs":dbl, "StopTimeNs":dbl, "Data Points":i32, "Compensation(ohm)":dbl, "DataFormat":i16, "Impedance Filter":bool, "Filter Risetime(ps)":dbl, "Impedance Spec String":string, "Skew Spec(ps)":i32, "CMP Setting":string}
  T10 = cluster{"Frequency(Hz)":dbl[], "output array":dbl[]}
  T11 = cluster{"Time Array":dbl[], "Impedance Data":dbl[]}
  T12 = cluster{"Time Array":dbl[], "Lower Spec":dbl[]}[]
  T13 = cluster{"Frequency(Hz)":dbl[], "lowerLimit":dbl[]}[]
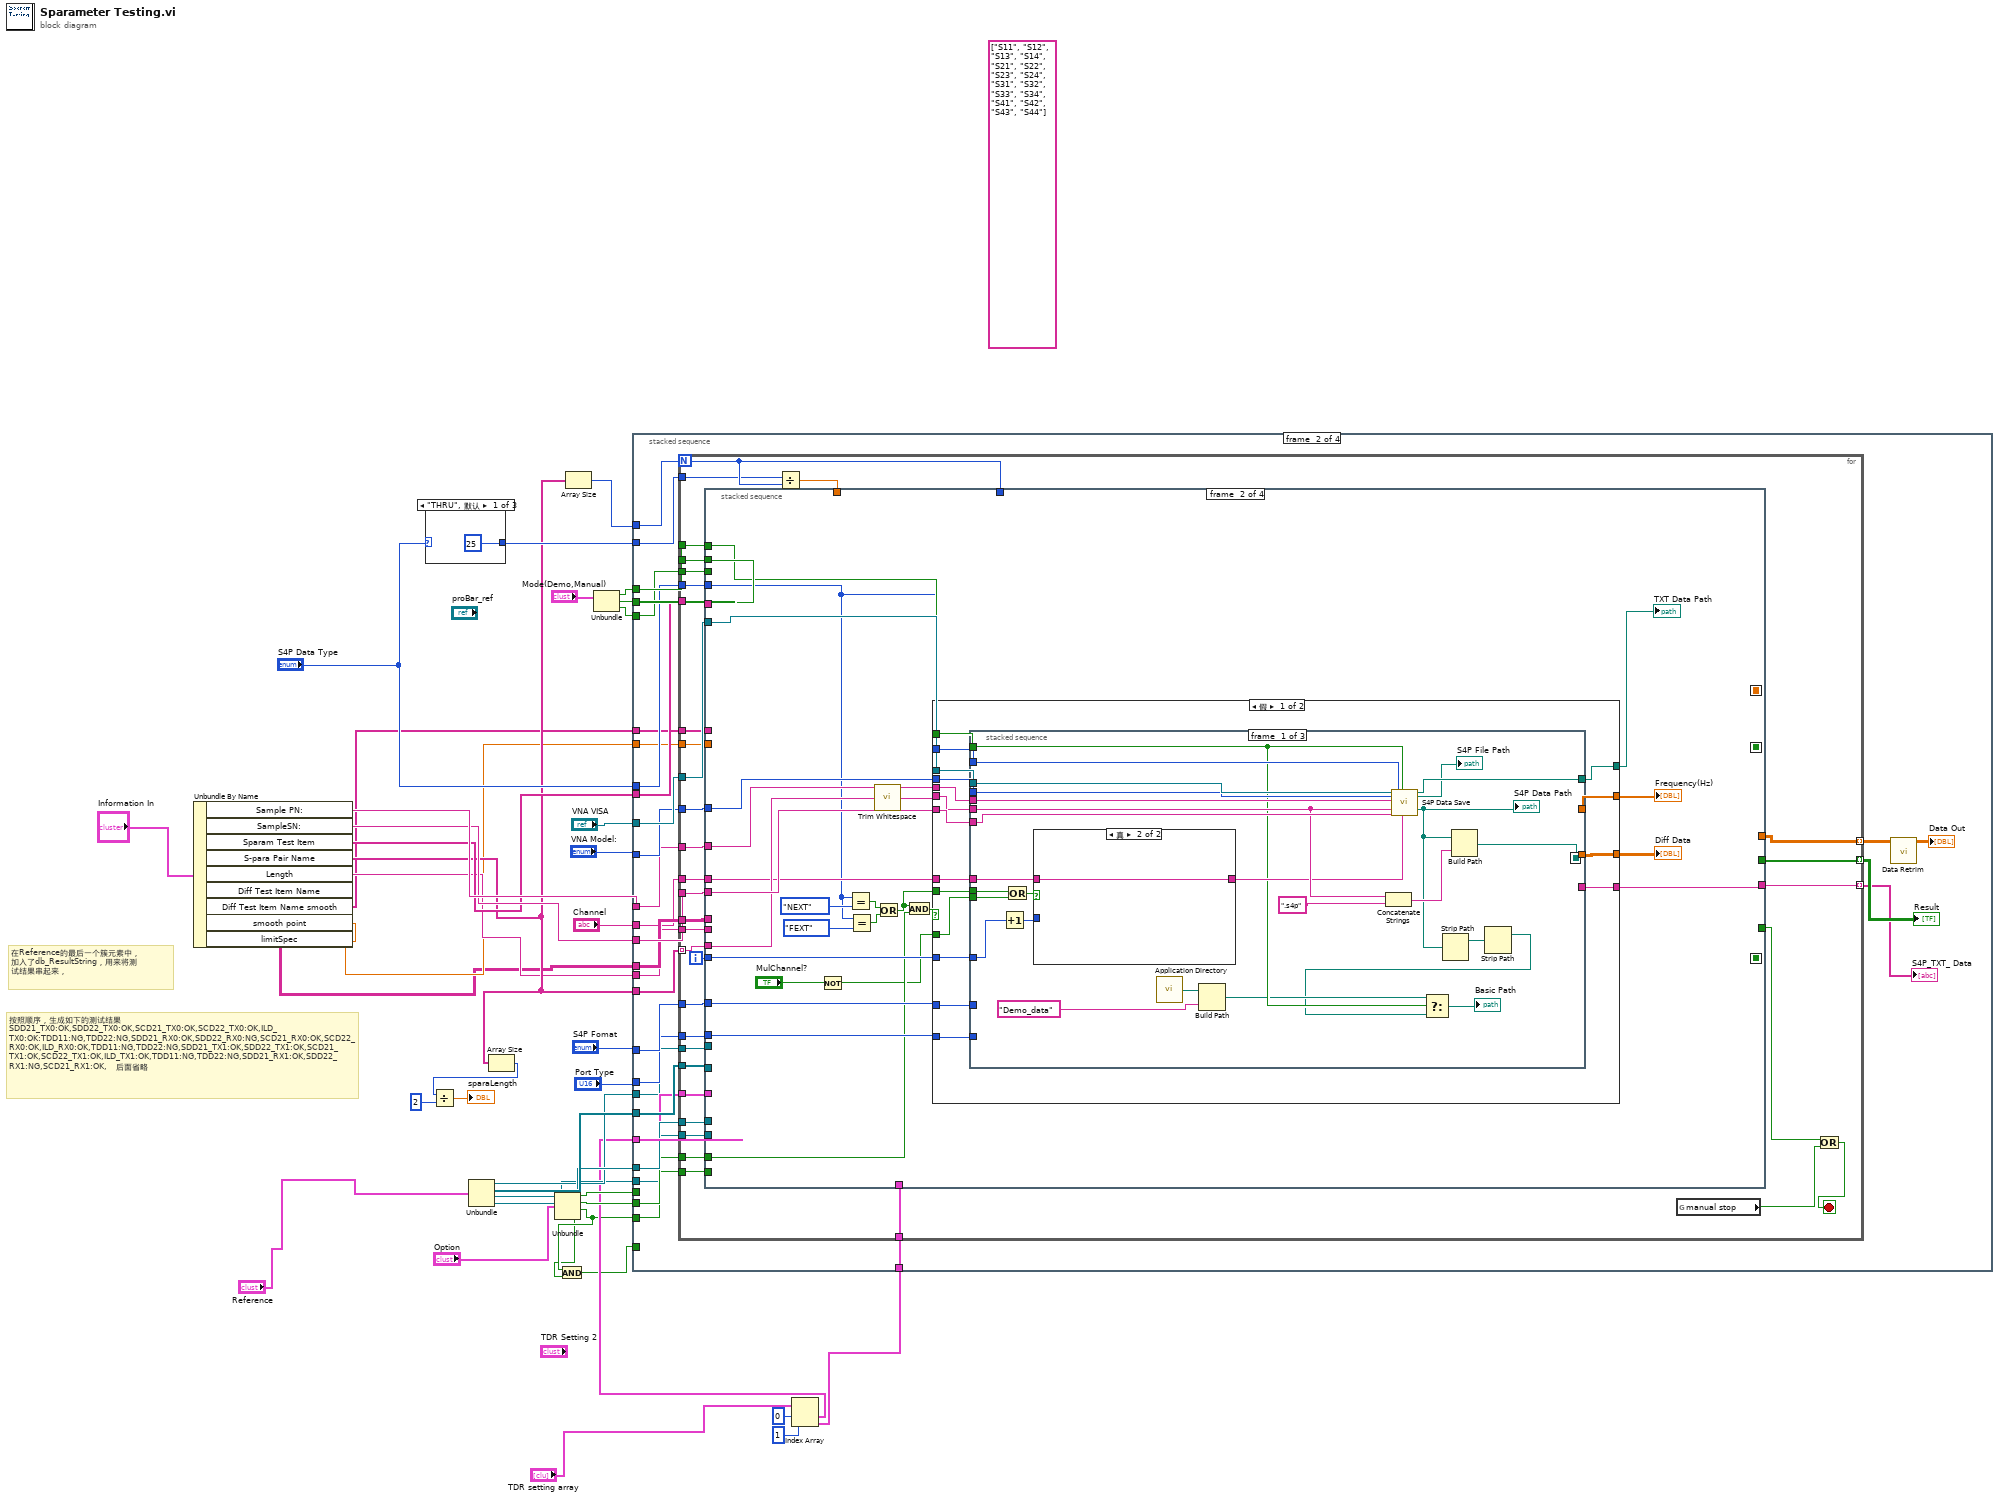
[diagram p0: block diagram]
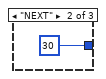
[diagram p2: hidden frame]
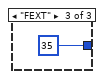
[diagram p3: hidden frame]
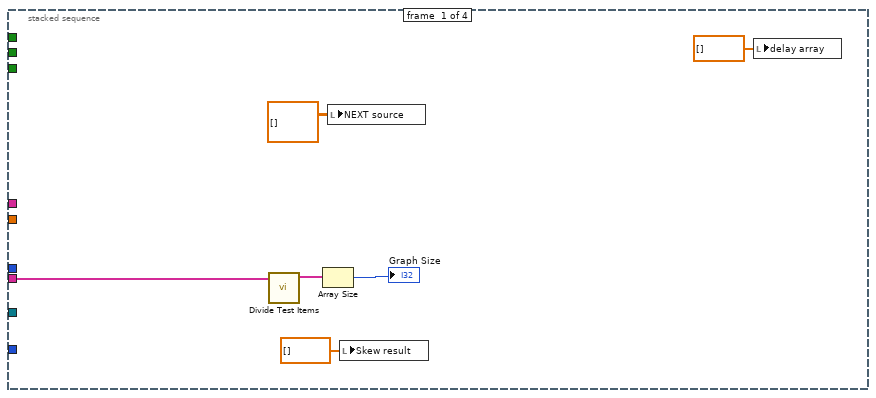
[diagram p4: hidden frame]
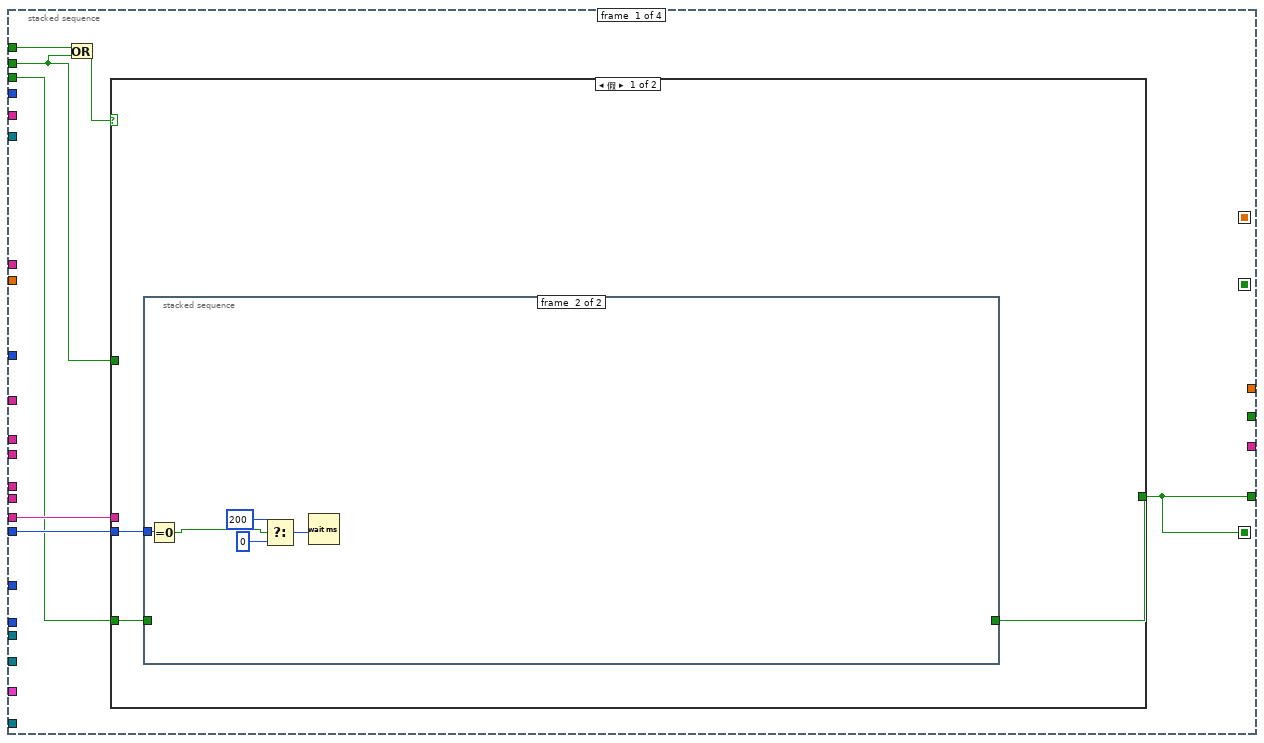
[diagram p5: hidden frame]
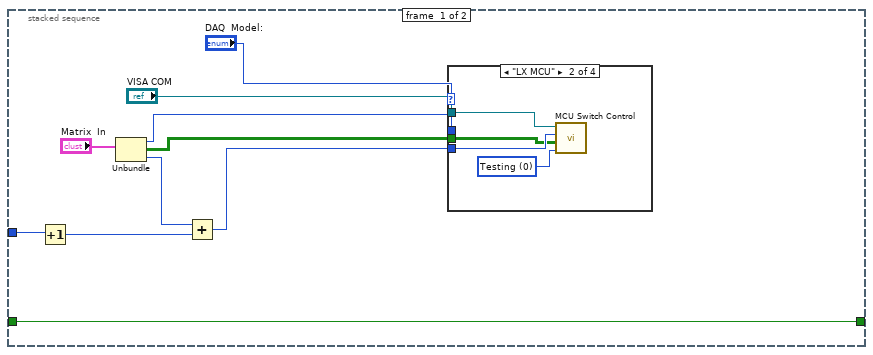
[diagram p6: hidden frame]
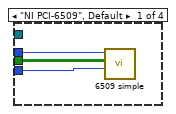
[diagram p7: hidden frame]
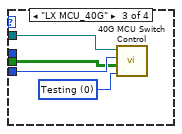
[diagram p8: hidden frame]
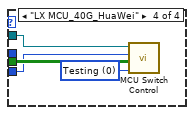
[diagram p9: hidden frame]
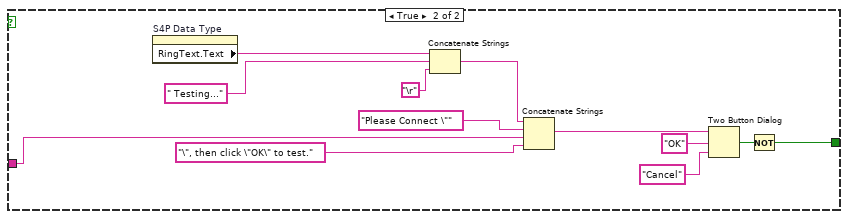
[diagram p11: hidden frame]
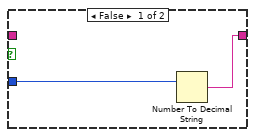
[diagram p12: hidden frame]
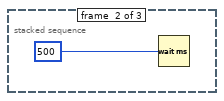
[diagram p13: hidden frame]
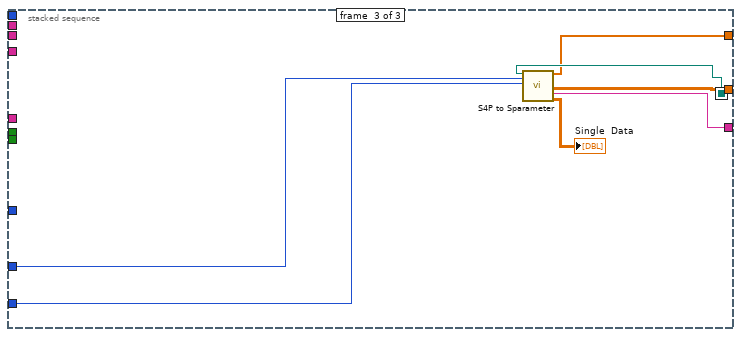
[diagram p14: hidden frame]
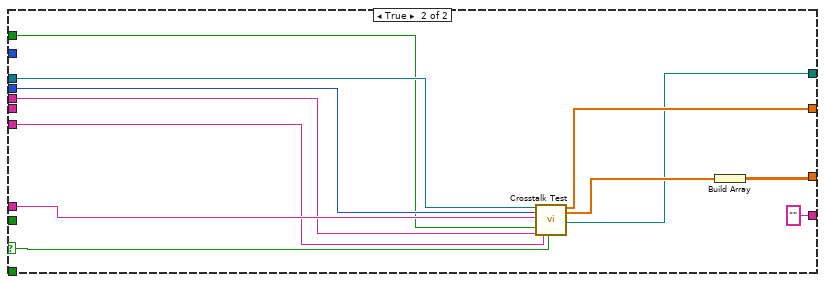
[diagram p15: hidden frame]
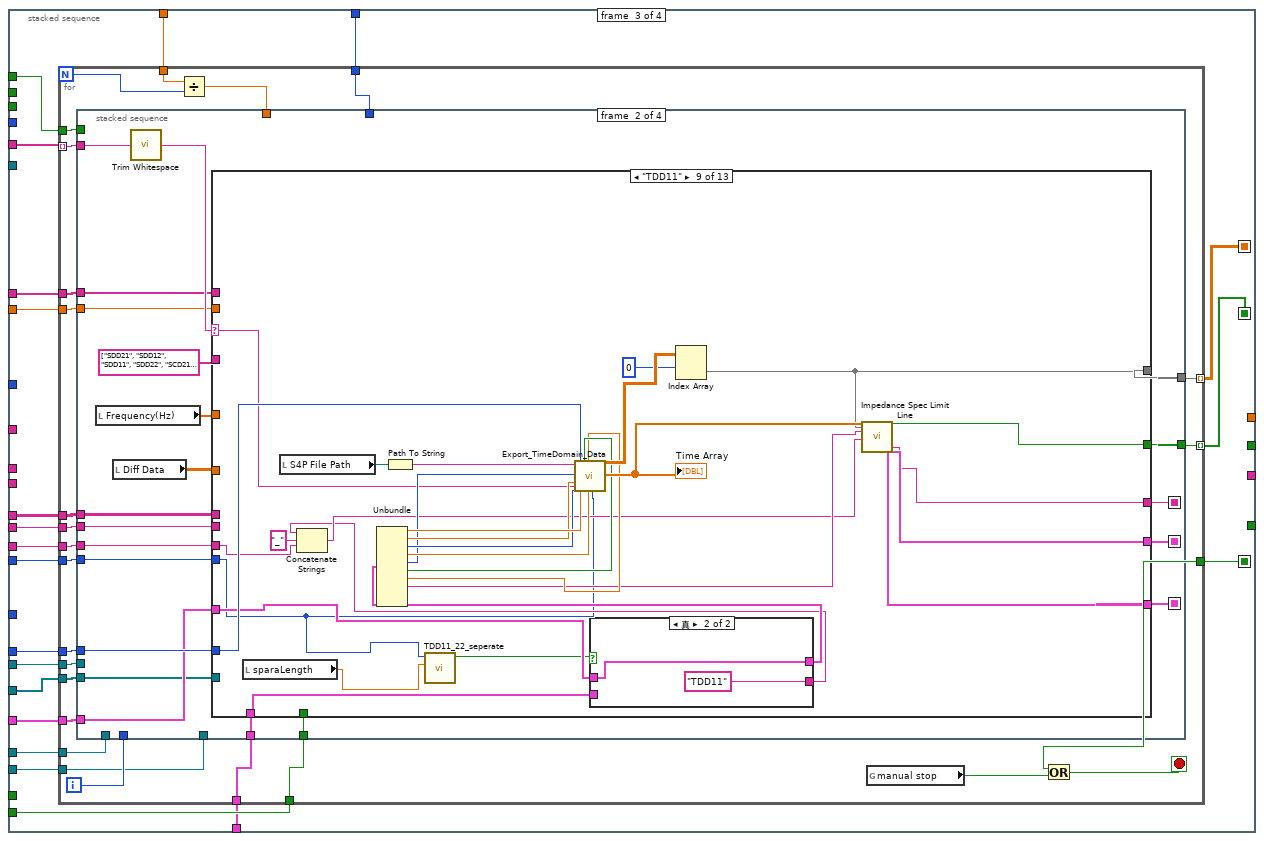
[diagram p16: hidden frame]
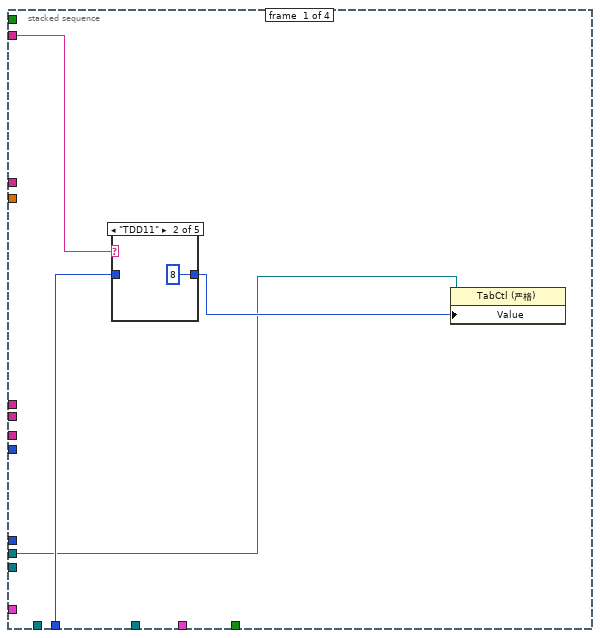
[diagram p17: hidden frame]
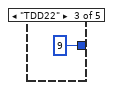
[diagram p19: hidden frame]
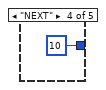
[diagram p20: hidden frame]
diagram:
  (unwired) string[] ["S11", "S12", "S13", "S14", "S21", "S22", "S23", "S24", "S31", "S32", "S33", "S34", "S41", "S42", "S43", "S44"]
  # "按照顺序，生成如下的测试结果\nSDD21_TX0:OK,SDD22_TX0:OK,SCD21_TX0:OK,SCD22_TX0:OK,ILD_TX0:OK:TDD11:NG,TDD22:NG,SDD21_RX0:OK,SDD22_RX0:NG,SCD21_RX0:OK,SCD22_RX0:OK,ILD_RX0:OK,TDD11:NG,TDD22:NG,SDD21_TX1:OK,SDD22_TX1:OK,SCD21_TX1:OK,SCD22_TX1:OK,ILD_TX1:OK,TDD11:NG,TDD22:NG,SDD21_RX1:OK,SDD22_RX1:NG,SCD21_RX1:OK,   后面省略"
  # "在Reference的最后一个簇元素中，\n加入了db_ResultString，用来将测\n试结果串起来，"
  n1 = Unbundle By Name("Information In") -> ("Sample PN:"=w8:string, "SampleSN:"=w7:string, "Sparam Test Item"=w6:string[], "S-para Pair Name"=w5:string[], "Length"=w4:string, "Diff Test Item Name smooth"=w3:string[], "smooth point"=w2:dbl, "limitSpec"=w1:string[][])  [unwired: 1 out]
  n2 = case shown="\"THRU\", 默认" "S4P Data Type" {
    tunnel: [u8 25 ("数值") u8 30 ("数值") u8 35 ("数值")] -> w23
    frame "THRU", Default {
    }
    frame "NEXT" {
    }
    frame "FEXT" {
    }
  }
  n3 = Unbundle("Reference") -> ("Tab_Graph"=w33:refnum<vi>, "Test Graph"=w35:refnum<vi>[], "Test Status:"=w34:refnum<vi>, "db_ResultString"=w24:refnum<vi>)
  n4 = Array Size(array=w5) -> (size(s)=w18:i32)
  n5 = Divide(x=w18, y=2) -> (x/y=→"sparaLength":dbl)
  n6 = Unbundle("Option") -> ("Data Convertion"=w26:bool, "Next by Trace"=w25:bool, "Dembel 2X"=w14:bool, "2X equalize"=w13:bool)
  n7 = And(x=w14, y=w13) -> (x .and. y?=w12:bool)
  n8 = Array Size(array=w5) -> (size(s)=w36:i32)
  n9 = Unbundle("Mode(Demo,Manual)") -> ("Demo Mode"=w31:bool, "Manual Mode"=w30:bool, "Urgent Stop"=w28:bool)
  n10 = Index Array(array="TDR setting array", index #1=0 ("索引"), index #2=1 ("索引")) -> (element #1=w20:T9, element #2=w19:T9)
  n11 = stacked-sequence {
    tunnel: w36 -> [_ w80 _ _]
    tunnel: w6 -> [w49 w79 w812 _]
    tunnel: "VNA VISA" -> [_ w78 _ _]
    tunnel: "VNA Model:" -> [_ w77 w801 _]
    tunnel: w8 -> [_ w76 _ _]
    tunnel: w7 -> [_ w75 _ _]
    tunnel: w31 -> [_ w74 _ _]
    tunnel: w5 -> [_ w73 _ _]
    tunnel: "S4P Fomat" -> [_ w72 _ _]
    tunnel: "Port Type" -> [_ w71 _ _]
    tunnel: w35 -> [_ w70 w794 _]
    tunnel: w1 -> [_ w69 _ _]
    tunnel: w34 -> [_ w67 w810 _]
    tunnel: w20 -> [_ w65 _ _]
    tunnel: "S4P Data Type" -> [_ w64 _ _]
    tunnel: w30 -> [_ w63 _ _]
    tunnel: w33 -> [_ w62 _ _]
    tunnel: w4 -> [_ w60 _ _]
    tunnel: "Channel" -> [_ w59 _ _]
    tunnel: w28 -> [_ w58 _ _]
    tunnel: w26 -> [_ _ _ w959]
    tunnel: w25 -> [_ w57 _ _]
    tunnel: w14 -> [_ w56 _ _]
    tunnel: w24 -> [_ w55 _ _]
    tunnel: w23 -> [_ w54 _ _]
    tunnel: w19 -> [_ w53 _ _]
    tunnel: w2 -> [_ w51 _ _]
    tunnel: w3 -> [_ w50 _ _]
    tunnel: w12 -> [_ _ w795 _]
    frame #0 {
      n12 = call "Divide Test Items.vi"("Test Item Name"=w49) -> ("S-Para Item List"=w48:string[])  [unwired: 9 in, 1 out]
      n13 = Array Size(array=w48) -> (size(s)=→"Graph Size":i32)
      n14 = local write "NEXT source"(dbl[][] [] ("NEXT source")) -> ()
      n15 = local write "Skew result"(dbl[] [] ("Skew result")) -> ()
      n16 = local write "delay array"(dbl[] [] ("delay array")) -> ()
    }
    frame #1 {
      n17 = for {
        N: w80 -> [w90]
        tunnel: w79 -> [w115]
        tunnel: w78 -> [w114]
        tunnel: w77 -> [w113]
        tunnel: w76 -> [w112]
        tunnel: w75 -> [w111]
        tunnel: w74 -> [w110]
        tunnel: w73 -> [w108] mode=indexing
        tunnel: w72 -> [w107]
        tunnel: w71 -> [w106]
        tunnel: w70 -> [w105]
        tunnel: w69 -> [w104]
        tunnel: [w103] -> w68 mode=indexing
        tunnel: w67 -> [w102]
        tunnel: w65 -> [w101]
        tunnel: w64 -> [w100]
        tunnel: w63 -> [w99]
        tunnel: w62 -> [w98]
        tunnel: [w97] -> w61 mode=indexing
        tunnel: w60 -> [w96]
        tunnel: w59 -> [w95]
        tunnel: w58 -> [w94]
        tunnel: w57 -> [w93]
        tunnel: w56 -> [w92]
        tunnel: w55 -> [w91]
        tunnel: w54 -> [w89]
        tunnel: w53 -> [w87]
        tunnel: [w86] -> w52 mode=indexing
        tunnel: w51 -> [w82]
        tunnel: w50 -> [w81]
        i -> [w109]
        stop <- w83 stop-if-true
        n18 = Divide(x=w89, y=w90) -> (x/y=w88:dbl)
        n19 = stacked-sequence {
          seq-local: [w117 _ _ _] -> [_ _ w274 _]
          seq-local: [_ _ w267 _] -> [_ _ _ w767]
          seq-local: [_ _ w266 _] -> [_ _ _ w764]
          tunnel: w115 -> [_ _ w269 w766]
          tunnel: w114 -> [_ w197 _ _]
          tunnel: w113 -> [_ w196 _ _]
          tunnel: w112 -> [_ w195 _ _]
          tunnel: w111 -> [_ w194 _ _]
          tunnel: w110 -> [w119 w187 w277 _]
          tunnel: w109 -> [w122 w185 w284 w761]
          tunnel: w108 -> [w120 w193 w283 _]
          tunnel: w107 -> [_ w192 _ _]
          tunnel: w106 -> [_ w191 w280 _]
          tunnel: w105 -> [_ _ w278 _]
          tunnel: w104 -> [_ _ w282 _]
          tunnel: [_ _ _ w763] -> w103
          tunnel: w102 -> [_ _ w281 _]
          tunnel: w101 -> [_ _ w279 _]
          tunnel: w100 -> [_ w181 _ _]
          tunnel: w99 -> [w118 _ _ _]
          tunnel: w98 -> [_ _ w276 _]
          tunnel: [_ w190 _ _] -> w97
          tunnel: w90 -> [_ _ w275 _]
          tunnel: [w117 _ _ _] -> w85
          tunnel: w96 -> [_ _ w273 _]
          tunnel: w95 -> [_ w189 _ _]
          tunnel: w94 -> [w116 _ _ _]
          tunnel: w93 -> [_ w178 _ _]
          tunnel: w92 -> [_ _ w272 _]
          tunnel: w91 -> [_ _ w271 _]
          tunnel: w88 -> [_ _ w270 _]
          tunnel: w87 -> [_ _ w268 _]
          tunnel: [_ _ _ w765] -> w86
          tunnel: w82 -> [_ _ w265 _]
          tunnel: w81 -> [_ _ w264 _]
          frame #0 {
            n20 = Or(x=w119, y=w118) -> (x .or. y?=w121:bool)
            n21 = case shown="假" w121 {
              tunnel: w122 -> [w125 _]
              tunnel: w118 -> [_ w159]
              tunnel: w120 -> [_ w158]
              tunnel: [w123 w157] -> w117
              tunnel: w116 -> [w124 w156]
              frame False {
                n22 = stacked-sequence {
                  tunnel: w125 -> [w130 w155]
                  tunnel: w124 -> [w126 _]
                  tunnel: [w126 _] -> w123
                  frame #0 {
                    n23 = Increment(x=w130) -> (x+1=w129:i32)
                    n24 = Unbundle("Matrix  In") -> ("DAQ device"=w134:enum16{"Dev1", "Dev2", "Dev3"}, "Matrix  In"=w131:bool[][], w133:i32)
                    n25 = Add(x=w133, y=w129) -> (x+y=w132:i32)
                    n26 = case shown="\"LX MCU\"" "DAQ  Model:" {
                      tunnel: w134 -> [w138 _ _ _]
                      tunnel: w132 -> [w137 w141 w145 w148]
                      tunnel: w131 -> [w136 w140 w144 w149]
                      tunnel: "VISA COM" -> [_ w142 w146 w150]
                      frame "NI PCI-6509", Default {
                        n27 = call "6509 simple.vi"("index (row)"=w137, "array input: P0-P1-P2-P3-P4-P5"=w136, "DAQ device"=w138) -> ()  [unwired: 4 in, 1 out]
                      }
                      frame "LX MCU" {
                        w139 = u16 0 items=["Testing", "Close All"] ("Function")
                        n28 = call "MCU Switch Control.vi"("Function"=w139, "Array input:"=w140, "Index"=w141, "VISA"=w142) -> ()  [unwired: 7 in, 1 out]
                      }
                      frame "LX MCU_40G" {
                        w143 = u16 0 items=["Testing", "Close All"] ("Function")
                        n29 = call "40G MCU Switch Control.vi"("Function"=w143, "Array input:"=w144, "Index"=w145, "VISA"=w146) -> ()  [unwired: 7 in, 1 out]
                      }
                      frame "LX MCU_40G_HuaWei" {
                        w147 = u16 0 items=["Testing", "Close All"] ("Function")
                        n30 = call "MCU Switch Control.vi"("Function"=w147, "Array input:"=w149, "Index"=w148, "VISA"=w150) -> ()  [unwired: 7 in, 1 out]
                      }
                    }
                  }
                  frame #1 {
                    n31 = Equal To 0?(x=w155) -> (x = 0?=w154:bool)
                    n32 = Select(t=200, s=w154, f=0) -> (s? t:f=w151:i32)
                    n33 = Wait (ms)(milliseconds to wait=w151) -> ()  [unwired: 1 out]
                  }
                }
              }
              frame True {
                n34 = case shown="假" w159 {
                  tunnel: w158 -> [_ w170]
                  tunnel: [w160 w161] -> w157
                  tunnel: w156 -> [w160 _]
                  frame False {
                  }
                  frame True {
                    n35 = property on="S4P Data Type" class="Enum (严格)"() -> ("RingText.Text"=w168:string)  [unwired: 2 in, 2 out]
                    n36 = Concatenate Strings(w168, " Testing..." ("字符串"), "\r") -> (w165:string)
                    n37 = Concatenate Strings(w165, "Please Connect \"" ("字符串"), w170, "\", then click \"OK\" to test." ("字符串")) -> (w172:string)
                    n38 = Two Button Dialog(message=w172, 1:"Cancel" ("F按钮名称（“取消”）"), 2:"OK" ("按钮名称（“确定”）")) -> (T button?=w162:bool)
                    n39 = Not(x=w162) -> (.not. x?=w161:bool)
                  }
                }
              }
            }
          }
          frame #1 {
            n40 = Not(x="MulChannel?") -> (.not. x?=w173:bool)
            n41 = Equal?(x=w181, y=enum16{"THRU", "NEXT", "FEXT"}."NEXT") -> (x = y?=w179:bool)
            n42 = Equal?(x=w181, y=enum16{"THRU", "NEXT", "FEXT"}."FEXT") -> (x = y?=w180:bool)
            n43 = call <vilib>:"Trim Whitespace.vi"("string"=w193) -> ("trimmed string"=w176:string)  [unwired: 1 in]
            n44 = Or(x=w179, y=w180) -> (x .or. y?=w174:bool)
            n45 = And(x=w174, y=w178) -> (x .and. y?=w186:bool)
            n46 = case shown="假" w186 {
              selector: w186 -> [_ w252]
              tunnel: w197 -> [w214 w262]
              tunnel: w196 -> [w213 w261]
              tunnel: w195 -> [w212 w255]
              tunnel: w194 -> [w211 w254]
              tunnel: w176 -> [w207 _]
              tunnel: w192 -> [w199 _]
              tunnel: w191 -> [w198 _]
              tunnel: [w200 "" ("TXT_Data")] -> w190
              tunnel: w189 -> [w204 w260]
              tunnel: w181 -> [w210 _]
              tunnel: w187 -> [w209 w259]
              tunnel: w185 -> [w203 _]
              tunnel: [w201 w257] -> w184
              tunnel: [w202 w256] -> w183
              tunnel: [w208 w253] -> w177
              tunnel: w174 -> [w206 _]
              tunnel: w173 -> [w205 _]
              frame False {
                n47 = stacked-sequence {
                  seq-local: [w221 _ _] -> [_ _ w250]
                  tunnel: w214 -> [w240 _ _]
                  tunnel: w213 -> [w239 _ _]
                  tunnel: w212 -> [w238 _ _]
                  tunnel: w211 -> [w237 _ _]
                  tunnel: w210 -> [w236 _ _]
                  tunnel: w209 -> [w218 _ _]
                  tunnel: [w235 _ _] -> w208
                  tunnel: w207 -> [w233 _ _]
                  tunnel: w206 -> [w229 _ _]
                  tunnel: w205 -> [w228 _ _]
                  tunnel: w204 -> [w227 _ _]
                  tunnel: w203 -> [w225 _ _]
                  tunnel: [_ _ w249] -> w202
                  tunnel: [_ _ w248] -> w201
                  tunnel: [_ _ w247] -> w200
                  tunnel: w199 -> [_ _ w246]
                  tunnel: w198 -> [_ _ w245]
                  frame #0 {
                    n48 = Increment(x=w225) -> (x+1=w224:i32)
                    n49 = Or(x=w229, y=w228) -> (x .or. y?=w230:bool)
                    n50 = case shown="真" w230 {
                      tunnel: w227 -> [_ w243]
                      tunnel: [w241 w243] -> w226
                      tunnel: w224 -> [w242 _]
                      frame False {
                        n51 = Number To Decimal String(number=w242) -> (decimal integer string=w241:string)  [unwired: 1 in]
                      }
                      frame True {
                      }
                    }
                    n52 = call <vilib>:"Application Directory.vi"() -> ("Application Directory"=w219:path)
                    n53 = Build Path(base path=w219, name or relative path="Demo_data" ("名称或相对路径")) -> (appended path=w217:path)
                    n54 = Concatenate Strings(w233, ".s4p" ("字符串")) -> (w231:string)
                    n55 = call "S4P Data Save.vi"("VNA VISA"=w240, "VNA Model:"=w239, "Sample PN:"=w238, "Pair  Name:"=w233, "SampleSN:"=w237, "S4P Data Type"=w236, "Demo Mode"=w218, "Channel"=w226) -> ("TXT Data Path"=w235:path, "S4P File Path"=→"S4P File Path":path, "S4P Data Path"=w223:path)  [unwired: 9 in]
                    "S4P Data Path" <- w223
                    n56 = Strip Path(path=w223) -> (stripped path=w222:path)  [unwired: 1 out]
                    n57 = Build Path(base path=w223, name or relative path=w231) -> (appended path=w221:path)
                    n58 = Strip Path(path=w222) -> (stripped path=w215:path)  [unwired: 1 out]
                    n59 = Select(t=w217, s=w218, f=w215) -> (s? t:f=→"Basic Path":path)
                  }
                  frame #1 {
                    n60 = Wait (ms)(milliseconds to wait=u32 500 ("等待时间（毫秒）")) -> ()  [unwired: 1 out]
                  }
                  frame #2 {
                    n61 = call "S4P to Sparameter.vi"("S4P File Path"=w250, "S4P Fomat"=w246, "Port Type"=w245) -> ("Frequency(Hz)"=w249:dbl[], "Diff S-parameters Data"=w248:dbl[][], "TXT_Data"=w247:string, "Single S-parameters Data"=→"Single  Data":dbl[][])  [unwired: 13 in]
                  }
                }
              }
              frame True {
                n62 = call "Crosstalk Test.vi"("VNA VISA"=w262, "VNA Model:"=w261, "Channel"=w260, "Demo Mode"=w259, "Sample PN:"=w255, "SampleSN:"=w254, "NEXT By Trace"=w252) -> ("Fre"=w256:dbl[], "Data out"=w258:dbl[], "dup path"=w253:path)  [unwired: 10 in]
                n63 = Build Array(w258) -> (w257:dbl[][])
              }
            }
            "Diff Data" <- w184
            "Frequency(Hz)" <- w183
            "TXT Data Path" <- w177
          }
          frame #2 {
            n64 = for {
              N -> [w293]
              tunnel: w269 -> [w310] mode=indexing
              tunnel: w284 -> [w301]
              tunnel: w283 -> [w309]
              tunnel: w282 -> [w308]
              tunnel: [w307] -> w266 mode=indexing
              tunnel: w281 -> [w300]
              tunnel: [w306] -> w267 mode=indexing
              tunnel: w280 -> [w304]
              tunnel: w279 -> [w303]
              tunnel: w278 -> [w302]
              tunnel: w277 -> [w299]
              tunnel: w276 -> [w298]
              tunnel: w275 -> [w297]
              tunnel: w274 -> [w289]
              tunnel: w273 -> [w296]
              tunnel: w272 -> [w295]
              tunnel: w271 -> [w294]
              tunnel: w270 -> [w292]
              tunnel: w268 -> [w290]
              tunnel: w265 -> [w286]
              tunnel: w264 -> [w285]
              i -> [w305]
              stop <- w287 stop-if-true
              n65 = Divide(x=w292, y=w293) -> (x/y=w291:dbl)
              n66 = stacked-sequence {
                seq-local: [_ w330 _ _] -> [_ _ w701 _]
                seq-local: [_ w329 _ _] -> [_ _ w700 _]
                seq-local: [_ w328 _ _] -> [_ _ w697 _]
                tunnel: w310 -> [w314 w326 w693 _]
                tunnel: w309 -> [_ w337 w698 _]
                tunnel: w308 -> [_ w336 _ _]
                tunnel: [_ w335 _ _] -> w307
                tunnel: [_ w334 _ _] -> w306
                tunnel: w305 -> [w313 _ w692 _]
                tunnel: w304 -> [_ w333 _ _]
                tunnel: w303 -> [_ w332 _ _]
                tunnel: w302 -> [_ w331 w702 _]
                tunnel: w301 -> [_ w324 w691 _]
                tunnel: w300 -> [_ _ w699 _]
                tunnel: w299 -> [_ _ _ _]
                tunnel: w298 -> [w311 _ _ _]
                tunnel: w297 -> [_ _ w695 _]
                tunnel: w296 -> [_ w327 _ _]
                tunnel: w295 -> [_ w323 _ _]
                tunnel: w294 -> [_ _ w696 _]
                tunnel: w291 -> [_ _ w694 _]
                tunnel: w290 -> [_ w322 _ _]
                tunnel: w286 -> [_ w321 _ _]
                tunnel: w285 -> [_ w320 _ _]
                frame #0 {
                  n67 = case shown="\"TDD11\"" w314 {
                    tunnel: w313 -> [w315 _ _ _ _]
                    tunnel: [w315 8 9 10 11] -> w312
                    frame "SDD21", Default {
                    }
                    frame "TDD11" {
                    }
                    frame "TDD22" {
                    }
                    frame "NEXT" {
                    }
                    frame "FEXT" {
                    }
                  }
                  n68 = property class="TabCtl (严格)"(reference=w311, "Value"=w312) -> ()  [unwired: 1 in, 2 out]
                }
                frame #1 {
                  n69 = local read "Frequency(Hz)"() -> (w338:dbl[])
                  n70 = local read "Diff Data"() -> (w340:dbl[][])
                  n71 = call <vilib>:"Trim Whitespace.vi"("string"=w326) -> ("trimmed string"=w325:string)  [unwired: 1 in]
                  n72 = case shown="\"TDD11\"" w325 {
                    selector: w325 -> [w344 w359 w376 w402 w433 w453 w468 w503 w542 w569 w607 w644 _]
                    tunnel: w340 -> [w353 w362 w392 w424 w446 w463 _ _ _ _ _ _ _]
                    tunnel: string[] ["SDD21", "SDD12", "SDD11", "SDD22", "SCD21", "SCD12", "SCD22", "SCD11", "SDC11", "SDC22", "SDC12", "SDC21", "SCC11", "SCC22", "SCC12", "SCC21"] ("字符串[]") -> [w355 w372 w394 w415 _ _ _ _ _ _ _ _ _]
                    tunnel: w338 -> [w350 w368 w389 w421 w437 w460 w466 w501 _ _ _ _ _]
                    tunnel: w337 -> [w352 w370 w391 w423 w445 w462 w473 w508 w541 w576 w614 w643 w671]
                    tunnel: w336 -> [w351 w369 w390 w422 w444 w461 w474 w509 _ _ _ _ _]
                    tunnel: [w341 w367 w388 w420 w443 w459 w470 w505 w556 w588 w624 w658 w672] -> w335
                    tunnel: [w342 w356 w384 w400 w430 w449 w464 w499 w557 w589 w625 w659 w679] -> w334
                    tunnel: w333 -> [_ _ _ _ _ _ _ _ w561 w593 w629 w663 w685]
                    tunnel: w332 -> [_ _ _ _ _ _ _ _ w540 w572 w610 w641 w684]
                    tunnel: w331 -> [_ _ _ _ _ _ _ _ _ _ _ _ _]
                    tunnel: [w347 w364 w385 w417 w440 w456 w465 w500 w555 w587 w623 w657 _] -> w329
                    tunnel: [w348 w365 w386 w418 w441 w457 w472 w507 w554 w586 w622 w656 w674] -> w330
                    tunnel: [w349 w366 w387 w419 w442 w458 w471 w506 w553 w585 w621 w655 w670] -> w328
                    tunnel: w327 -> [_ _ _ _ _ _ _ _ _ _ _ _ w681]
                    tunnel: w324 -> [_ _ _ _ _ _ w481 w516 w535 w574 w612 w638 _]
                    tunnel: w323 -> [_ _ w381 w406 _ _ _ _ _ _ _ _ _]
                    tunnel: w322 -> [_ _ _ _ _ _ _ _ w539 w571 w609 w642 _]
                    tunnel: w321 -> [w346 w358 w375 w401 w432 w451 w467 w502 _ _ _ _ _]
                    tunnel: w320 -> [w345 w360 w377 w403 w434 w454 w469 w504 _ _ _ _ _]
                    frame "SDD22", Default {
                      n73 = Search 1D Array(1D array=w355, element=w344) -> (index of element=w354:i32)  [unwired: 1 in]
                      n74 = Index Array(array=w353, index (row)=w354) -> (element=w343:dbl[])  [unwired: 1 in]
                      n75 = call "smooth test data.vi"("smooth point"=w346, "input array"=w343, "test item name smooth"=w345, "test item name"=w344) -> ("output array"=w342:dbl[])  [unwired: 7 in]
                      n76 = Bundle("Frequency(Hz)"=w350, "output array"=w342) -> (w347:T10)  [unwired: 1 in]
                      n77 = call "SParam Limit Testing.vi"("Item Name"=w344, "Frequency"=w350, "Pair Name"=w352, "specData"=w351, "Data In"=w342) -> ("test passed?"=w341:bool, "Test Summary"=w349:string, "Limit Data"=w348:cluster{"Frequency":dbl[], "Data In":dbl[]}[])  [unwired: 11 in, 1 out]
                    }
                    frame "SCC11" {
                      n78 = Search 1D Array(1D array=w372, element=w359) -> (index of element=w371:i32)  [unwired: 1 in]
                      n79 = Index Array(array=w362, index (row)=w371) -> (element=w363:dbl[])  [unwired: 1 in]
                      n80 = Subtract(x=w363, y=0.9) -> (x-y=w357:dbl[])
                      n81 = call "smooth test data.vi"("smooth point"=w358, "input array"=w357, "test item name smooth"=w360, "test item name"=w359) -> ("output array"=w356:dbl[])  [unwired: 7 in]
                      n82 = Bundle("Frequency(Hz)"=w368, "output array"=w356) -> (w364:T10)  [unwired: 1 in]
                      n83 = call "SParam Limit Testing.vi"("Item Name"=w359, "Frequency"=w368, "Pair Name"=w370, "specData"=w369, "Data In"=w356) -> ("test passed?"=w367:bool, "Test Summary"=w366:string, "Limit Data"=w365:cluster{"Frequency":dbl[], "Data In":dbl[]}[])  [unwired: 11 in, 1 out]
                    }
                    frame "SDD21" {
                      n84 = Search 1D Array(1D array=w394, element=w376) -> (index of element=w393:i32)  [unwired: 1 in]
                      n85 = Index Array(array=w392, index (row)=w393) -> (element=w374:dbl[])  [unwired: 1 in]
                      n86 = Not Equal?(x="2X Thru", y=dbl[] []) -> (x != y?=w380:bool[])
                      n87 = call "smooth test data.vi"("smooth point"=w375, "input array"=w374, "test item name smooth"=w377, "test item name"=w376) -> ("output array"=w373:dbl[])  [unwired: 7 in]
                      n88 = And Array Elements(Boolean array=w380) -> (logical AND=w379:bool)
                      n89 = And(x=w381, y=w379) -> (x .and. y?=w382:bool)
                      n90 = case shown="真" w382 {
                        tunnel: w373 -> [w395 w398]
                        tunnel: [w395 w397] -> w384
                        tunnel: "2X Thru" -> [_ w396]
                        frame False {
                        }
                        frame True {
                          n91 = Subtract(x=w398, y=w396) -> (x-y=w397:dbl[])
                        }
                      }
                      n92 = call "SParam Limit Testing.vi"("Item Name"=w376, "Frequency"=w389, "Pair Name"=w391, "specData"=w390, "Data In"=w384) -> ("test passed?"=w388:bool, "Test Summary"=w387:string, "Limit Data"=w386:cluster{"Frequency":dbl[], "Data In":dbl[]}[])  [unwired: 11 in, 1 out]
                      n93 = Bundle("Frequency(Hz)"=w389, "output array"=w384) -> (w385:T10)  [unwired: 1 in]
                    }
                    frame "SCD21-SDD21" {
                      # "Add  when test scd21-sdd21 \n-2X value."
                      n94 = local read "2X Thru"() -> (w404:dbl[])
                      n95 = Search 1D Array(1D array=w415, element="SDD21" ("元素")) -> (index of element=w413:i32)  [unwired: 1 in]
                      n96 = Search 1D Array(1D array=w415, element="SCD21" ("元素")) -> (index of element=w425:i32)  [unwired: 1 in]
                      n97 = Index Array(array=w424, index (row) #1=w425, index (row) #2=w413) -> (element #1=w411:dbl[], element #2=w412:dbl[])  [unwired: 2 in]
                      n98 = Not Equal?(x=w404, y=dbl[] []) -> (x != y?=w408:bool[])
                      n99 = Subtract(x=w411, y=w412) -> (x-y=w405:dbl[])
                      n100 = And Array Elements(Boolean array=w408) -> (logical AND=w407:bool)
                      n101 = And(x=w406, y=w407) -> (x .and. y?=w409:bool)
                      n102 = case shown="真" w409 {
                        tunnel: w405 -> [w426 w429]
                        tunnel: [w426 w428] -> w399
                        tunnel: w404 -> [_ w427]
                        frame False {
                        }
                        frame True {
                          n103 = Add(x=w429, y=w427) -> (x+y=w428:dbl[])
                        }
                      }
                      n104 = call "smooth test data.vi"("smooth point"=w401, "input array"=w399, "test item name smooth"=w403, "test item name"=w402) -> ("output array"=w400:dbl[])  [unwired: 7 in]
                      n105 = Bundle("Frequency(Hz)"=w421, "output array"=w400) -> (w417:T10)  [unwired: 1 in]
                      n106 = call "SParam Limit Testing.vi"("Item Name"=w402, "Frequency"=w421, "Pair Name"=w423, "specData"=w422, "Data In"=w400) -> ("test passed?"=w420:bool, "Test Summary"=w419:string, "Limit Data"=w418:cluster{"Frequency":dbl[], "Data In":dbl[]}[])  [unwired: 11 in, 1 out]
                    }
                    frame "ILD", "ILD_15" {
                      n107 = Index Array(array=w446, index (row)=0 ("索引 (行)")) -> (element=w436:dbl[])  [unwired: 1 in]
                      n108 = call "ILD from Array Data.vi"("Frequency"=w437, "Data in"=w436, "Spec"="ILDSpec") -> ("Size"=→"Size":i32, "ILD Data"=w431:dbl[])  [unwired: 5 in, 2 out]
                      n109 = call "smooth test data.vi"("smooth point"=w432, "input array"=w431, "test item name smooth"=w434, "test item name"=w433) -> ("output array"=w430:dbl[])  [unwired: 7 in]
                      n110 = Bundle("Frequency(Hz)"=w437, "output array"=w430) -> (w440:T10)  [unwired: 1 in]
                      n111 = call "SParam Limit Testing.vi"("Item Name"=w433, "Frequency"=w437, "Pair Name"=w445, "specData"=w444, "Data In"=w430) -> ("test passed?"=w443:bool, "Test Summary"=w442:string, "Limit Data"=w441:cluster{"Frequency":dbl[], "Data In":dbl[]}[])  [unwired: 11 in, 1 out]
                    }
                    frame "FEXT", "NEXT" {
                      n112 = Index Array(array=w463, index (row)=0 ("索引 (行)")) -> (element=w452:dbl[])  [unwired: 1 in]
                      n113 = call "smooth test data.vi"("smooth point"=w451, "input array"=w452, "test item name smooth"=w454, "test item name"=w453) -> ("output array"=w449:dbl[])  [unwired: 7 in]
                      "smoothed Diff Data" <- w449
                      n114 = Bundle("Frequency(Hz)"=w460, "output array"=w449) -> (w456:T10)  [unwired: 1 in]
                      n115 = call "SParam Limit Testing.vi"("Item Name"=w453, "Frequency"=w460, "Pair Name"=w462, "specData"=w461, "Data In"=w449) -> ("test passed?"=w459:bool, "Test Summary"=w458:string, "Limit Data"=w457:cluster{"Frequency":dbl[], "Data In":dbl[]}[])  [unwired: 11 in, 1 out]
                      n116 = Insert Into Array(array="NEXT source", new element=w449) -> (w448:dbl[][])  [unwired: 2 in]
                      n117 = local write "NEXT source"(w448) -> ()
                      n118 = Transpose 2D Array(2D array=w448) -> (transposed array=→"NextSourced":dbl[][])
                    }
                    frame "MDNEXT" {
                      n119 = Increment(x=w481) -> (x+1=w480:i32)
                      n120 = Quotient & Remainder(x=w480, y=4) -> (x-y*floor(x/y)=w478:i32, floor(x/y)=w476:i32)
                      n121 = Decrement(x=w476) -> (x-1=w475:i32)
                      n122 = Equal To 0?(x=w478) -> (x = 0?=w477:bool)
                      n123 = case shown="真" w477 {
                        tunnel: w475 -> [_ w483]
                        tunnel: w466 -> [_ w498]
                        tunnel: w474 -> [_ w497]
                        tunnel: w468 -> [_ w496]
                        tunnel: w473 -> [_ w495]
                        tunnel: [_ w494] -> w472
                        tunnel: [_ w493] -> w471
                        tunnel: [TRUE ("test passed?") w492] -> w470
                        tunnel: w469 -> [_ w491]
                        tunnel: w468 -> [_ w490]
                        tunnel: w467 -> [_ w489]
                        tunnel: w466 -> [_ w487]
                        tunnel: [_ w486] -> w465
                        tunnel: [_ w485] -> w464
                        frame False {
                        }
                        frame True {
                          n124 = local read "NextSourced"() -> (w484:dbl[][])
                          n125 = call "MDNEXT.vi"("index"=w483, "NextSource"=w484) -> ("MDNext"=w488:dbl[])  [unwired: 9 in]
                          n126 = call "smooth test data.vi"("smooth point"=w489, "input array"=w488, "test item name smooth"=w491, "test item name"=w490) -> ("output array"=w485:dbl[])  [unwired: 7 in]
                          n127 = Bundle("Frequency(Hz)"=w487, "output array"=w485) -> (w486:T10)  [unwired: 1 in]
                          n128 = call "SParam Limit Testing.vi"("Item Name"=w496, "Frequency"=w498, "Pair Name"=w495, "specData"=w497, "Data In"=w485) -> ("test passed?"=w492:bool, "Test Summary"=w493:string, "Limit Data"=w494:cluster{"Frequency":dbl[], "Data In":dbl[]}[])  [unwired: 11 in, 1 out]
                        }
                      }
                    }
                    frame "MDFEXT" {
                      n129 = Increment(x=w516) -> (x+1=w515:i32)
                      n130 = Quotient & Remainder(x=w515, y=3) -> (x-y*floor(x/y)=w513:i32, floor(x/y)=w511:i32)
                      n131 = Decrement(x=w511) -> (x-1=w510:i32)
                      n132 = Equal To 0?(x=w513) -> (x = 0?=w512:bool)
                      n133 = case shown="真" w512 {
                        tunnel: w510 -> [_ w532]
                        tunnel: w501 -> [_ w531]
                        tunnel: w509 -> [_ w530]
                        tunnel: w503 -> [_ w529]
                        tunnel: w508 -> [_ w528]
                        tunnel: [_ w527] -> w507
                        tunnel: [_ w526] -> w506
                        tunnel: [TRUE ("test passed?") w525] -> w505
                        tunnel: w504 -> [_ w524]
                        tunnel: w503 -> [_ w523]
                        tunnel: w502 -> [_ w522]
                        tunnel: w501 -> [_ w520]
                        tunnel: [_ w519] -> w500
                        tunnel: [_ w518] -> w499
                        frame False {
                        }
                        frame True {
                          n134 = local read "NextSourced"() -> (w533:dbl[][])
                          n135 = call "MDFEXT.vi"("index"=w532, "NextSource"=w533) -> ("MDNext"=w521:dbl[])  [unwired: 9 in]
                          n136 = call "smooth test data.vi"("smooth point"=w522, "input array"=w521, "test item name smooth"=w524, "test item name"=w523) -> ("output array"=w518:dbl[])  [unwired: 7 in]
                          n137 = Bundle("Frequency(Hz)"=w520, "output array"=w518) -> (w519:T10)  [unwired: 1 in]
                          n138 = call "SParam Limit Testing.vi"("Item Name"=w529, "Frequency"=w531, "Pair Name"=w528, "specData"=w530, "Data In"=w518) -> ("test passed?"=w525:bool, "Test Summary"=w526:string, "Limit Data"=w527:cluster{"Frequency":dbl[], "Data In":dbl[]}[])  [unwired: 11 in, 1 out]
                        }
                      }
                    }
                    frame "TDD11" {
                      n139 = local read "sparaLength"() -> (w536:dbl)
                      n140 = local read "S4P File Path"() -> (w563:path)
                      n141 = Path To String(path=w563) -> (string=w562:string)
                      n142 = call "TDD11_22_seperate.vi"("paraLength"=w536, "pairIndex"=w535) -> ("is TDD11?"=w534:bool)  [unwired: 9 in]
                      n143 = case shown="真" w534 {
                        tunnel: w540 -> [_ w567]
                        tunnel: [w565 w567] -> w538
                        tunnel: w539 -> [w565 _]
                        tunnel: ["TDD22" "TDD11"] -> w537
                        frame False {
                        }
                        frame True {
                        }
                      }
                      n144 = Concatenate Strings(w537, "_" ("字符串"), w541) -> (w543:string)
                      n145 = Unbundle(w538) -> ("Start TimeNs"=w552:dbl, "StopTimeNs"=w551:dbl, "Data Points"=w550:i32, "Compensation(ohm)"=w549:dbl, "DataFormat"=w548:i16, "Impedance Filter"=w547:bool, "Filter Risetime(ps)"=w546:dbl, "Impedance Spec String"=w545:string)  [unwired: 2 out]
                      n146 = call "Export_TimeDomain_Data.vi"("szFileName"=w562, "dataFormat"=w548, "stopTimeNs"=w551, "ParamList"=w542, "Data Points"=w550, "Port Type"=w561, "startTimeNs"=w552, "Filter?"=w547, "Filter Risetime(ps)"=w546, "Compensation(ohm)"=w549, "Index"=w535) -> ("Data Out"=w560:dbl[][], "Time Array"=w558:dbl[])  [unwired: 15 in]
                      "Time Array" <- w558
                      n147 = Index Array(array=w560, index (row)=0 ("索引 (行)")) -> (element=w557:dbl[])  [unwired: 1 in]
                      n148 = call "Impedance Spec Limit Line.vi"("Time Array"=w558, "Impedance Data"=w557, "Impedance Spec String"=w545, "Des."=w543) -> ("Test Data"=w555:T11, "test passed?"=w556:bool, "Test Summary"=w553:string, "Impedance Chart"=w554:T12)  [unwired: 16 in, 4 out]
                    }
                    frame "TCC11", "TCC22" {
                      n149 = local read "sparaLength"() -> (w575:dbl)
                      n150 = local read "S4P File Path"() -> (w595:path)
                      n151 = Concatenate Strings(w569, "_" ("字符串"), w576) -> (w577:string)
                      n152 = Less?(x=w574, y=w575) -> (x < y?=w573:bool)
                      n153 = Path To String(path=w595) -> (string=w594:string)
                      n154 = case shown="假" w573 {
                        tunnel: w572 -> [w596 w599]
                        tunnel: [w596 w599] -> w570
                        tunnel: w571 -> [_ _]
                        tunnel: ["TDD22" "TDD11"] -> _
                        frame False {
                        }
                        frame True {
                        }
                      }
                      n155 = Unbundle(w570) -> ("Start TimeNs"=w584:dbl, "StopTimeNs"=w583:dbl, "Data Points"=w582:i32, "Compensation(ohm)"=w581:dbl, "DataFormat"=w580:i16, "Filter Risetime(ps)"=w579:dbl, "CMP Setting"=w568:string)  [unwired: 3 out]
                      n156 = call "Export_TimeDomain_Data.vi"("szFileName"=w594, "dataFormat"=w580, "stopTimeNs"=w583, "ParamList"=w569, "Data Points"=w582, "Port Type"=w593, "startTimeNs"=w584, "Filter Risetime(ps)"=w579, "Compensation(ohm)"=w581, "Index"=w574) -> ("Data Out"=w592:dbl[][], "Time Array"=w590:dbl[])  [unwired: 16 in]
                      "Time Array 3" <- w590
                      n157 = Index Array(array=w592, index (row)=0 ("索引 (行)")) -> (element=w589:dbl[])  [unwired: 1 in]
                      n158 = call "Impedance Spec Limit Line.vi"("Time Array"=w590, "Impedance Data"=w589, "Impedance Spec String"=w568, "Des."=w577) -> ("Test Data"=w587:T11, "test passed?"=w588:bool, "Test Summary"=w585:string, "Impedance Chart"=w586:T12)  [unwired: 16 in, 4 out]
                    }
                    frame "Delay" {
                      w606 = i16 2 items=["StepReal", "ImpulseReal", "StepVolts", "ImpulseVolts", "StepLog", "ImpulseLog", "StepImpedance"] ("dataFormat")
                      n159 = local read "sparaLength"() -> (w613:dbl)
                      n160 = local read "S4P File Path"() -> (w631:path)
                      n161 = Concatenate Strings(w607, "_" ("字符串"), w614) -> (w615:string)
                      n162 = Less?(x=w612, y=w613) -> (x < y?=w611:bool)
                      n163 = Path To String(path=w631) -> (string=w630:string)
                      n164 = case shown="真" w611 {
                        tunnel: w610 -> [w632 w635]
                        tunnel: [w632 w635] -> w608
                        tunnel: w609 -> [_ _]
                        tunnel: ["TDD22" "TDD11"] -> _
                        frame False {
                        }
                        frame True {
                        }
                      }
                      n165 = Unbundle(w608) -> ("Start TimeNs"=w620:dbl, "Data Points"=w619:i32, "Compensation(ohm)"=w618:dbl, "Filter Risetime(ps)"=w617:dbl)  [unwired: 6 out]
                      n166 = call "Export_TimeDomain_Data.vi"("szFileName"=w630, "dataFormat"=w606, "stopTimeNs"=53.0, "ParamList"="TDD21", "Data Points"=w619, "Port Type"=w629, "startTimeNs"=w620, "Filter Risetime(ps)"=w617, "Compensation(ohm)"=w618, "Index"=w612) -> ("Data Out"=w628:dbl[][], "Time Array"=w626:dbl[])  [unwired: 16 in]
                      "Time Array 4" <- w626
                      n167 = Index Array(array=w628, index (row)=0 ("索引 (行)")) -> (element=w625:dbl[])  [unwired: 1 in]
                      n168 = call "delay chart.vi"("Spec"=100.0, "Des."=w615, "Impedance Data"=w625, "Time Array"=w626) -> ("Test Summary"=w621:string, "test passed?"=w624:bool, "Test Data"=w623:T11, "Impedance Chart"=w622:T12, "delay"=w603:dbl)  [unwired: 3 in]
                      n169 = Insert Into Array(array="delay array", new element=w603) -> (w601:dbl[])  [unwired: 1 in]
                      n170 = local write "delay array"(w601) -> ()
                    }
                    frame "TDD22" {
                      n171 = local read "sparaLength"() -> (w637:dbl)
                      n172 = local read "S4P File Path"() -> (w665:path)
                      n173 = Path To String(path=w665) -> (string=w664:string)
                      n174 = call "TDD11_22_seperate.vi"("paraLength"=w637, "pairIndex"=w638) -> ("is TDD11?"=w636:bool)  [unwired: 9 in]
                      n175 = case shown="假" w636 {
                        tunnel: w642 -> [_ w669]
                        tunnel: [w667 w669] -> w640
                        tunnel: w641 -> [w667 _]
                        tunnel: ["TDD11" "TDD22"] -> w639
                        frame False {
                        }
                        frame True {
                        }
                      }
                      n176 = Concatenate Strings(w639, "_" ("字符串"), w643) -> (w645:string)
                      n177 = Unbundle(w640) -> ("Start TimeNs"=w654:dbl, "StopTimeNs"=w653:dbl, "Data Points"=w652:i32, "Compensation(ohm)"=w651:dbl, "DataFormat"=w650:i16, "Impedance Filter"=w649:bool, "Filter Risetime(ps)"=w648:dbl, "Impedance Spec String"=w647:string)  [unwired: 2 out]
                      n178 = call "Export_TimeDomain_Data.vi"("szFileName"=w664, "dataFormat"=w650, "stopTimeNs"=w653, "ParamList"=w644, "Data Points"=w652, "Port Type"=w663, "startTimeNs"=w654, "Filter?"=w649, "Filter Risetime(ps)"=w648, "Compensation(ohm)"=w651, "Index"=w638) -> ("Data Out"=w662:dbl[][], "Time Array"=w660:dbl[])  [unwired: 15 in]
                      "Time Array 2" <- w660
                      n179 = Index Array(array=w662, index (row)=0 ("索引 (行)")) -> (element=w659:dbl[])  [unwired: 1 in]
                      n180 = call "Impedance Spec Limit Line.vi"("Time Array"=w660, "Impedance Data"=w659, "Impedance Spec String"=w647, "Des."=w645) -> ("Test Data"=w657:T11, "test passed?"=w658:bool, "Test Summary"=w655:string, "Impedance Chart"=w656:T12)  [unwired: 16 in, 4 out]
                    }
                    frame "PSkew", "Pskew" {
                      n181 = Unbundle By Name(w684) -> ("Filter Risetime(ps)"=w683:dbl, "Impedance Filter"=w682:bool, "Skew Spec(ps)"=w673:i32)
                      n182 = Decimal String To Number(string=w681) -> (number=w680:i32)  [unwired: 2 in, 1 out]
                      n183 = local read "S4P File Path"() -> (w686:path)
                      n184 = call "Intra-pair Skew Test.vi"("Data path"=w686, "Port Type"=w685, "Length(mm)"=w680, "Skew Spec(ps)"=w673, "Filter Risetime(ps)"=w683, "Filter?"=w682, "Pair Name"=w671) -> ("Test Summay"=w670:string, "Dataout"=w679:dbl[], "Time Array"=→"Skew Time":dbl[], "Intra-pair Skew Value(ps)"=w677:dbl, "Skew Chart"=w674:cluster{"Time Array":dbl[], "Data Out":dbl[]}[], "Result"=w672:bool)  [unwired: 6 in, 1 out]
                      n185 = Insert Into Array(array="Skew result", new element=w677) -> (w675:dbl[])  [unwired: 1 in]
                      n186 = local write "Skew result"(w675) -> ()
                    }
                  }
                }
                frame #2 {
                  n187 = call <vilib>:"Trim Whitespace.vi"("string"=w693) -> ("trimmed string"=w689:string)  [unwired: 1 in]
                  n188 = To Upper Case(1:w689) -> (0:w688:string)
                  n189 = Equal?(x=w688, y="ILD_15") -> (x = y?=w687:bool)
                  n190 = case shown="假" w687 {
                    tunnel: w702 -> [w731 _]
                    tunnel: w701 -> [w730 _]
                    tunnel: w700 -> [w729 _]
                    tunnel: w699 -> [w728 _]
                    tunnel: w698 -> [w726 _]
                    tunnel: w697 -> [w723 _]
                    tunnel: w696 -> [w722 _]
                    tunnel: w695 -> [w712 _]
                    tunnel: w694 -> [w708 _]
                    tunnel: w689 -> [w707 _]
                    tunnel: w692 -> [w706 w758]
                    tunnel: w691 -> [w705 _]
                    frame False {
                      w714 = "," ("替换字符串(\"\")")
                      w727 = u16 0 items=["Normal Input", "Start", "Product Inf", "End"] ("Summary Method")
                      n191 = case shown="\"TDD22\"" w707 {
                        selector: w707 -> [w732 w738 w750]
                        tunnel: w706 -> [w733 w740 w752]
                        tunnel: w705 -> [_ w736 w747]
                        tunnel: [w733 w739 w751] -> w703
                        tunnel: [w732 w737 w749] -> w704
                        frame "假", Default {
                        }
                        frame "TDD11" {
                          n192 = local read "sparaLength"() -> (w735:dbl)
                          n193 = call "TDD11_22_seperate.vi"("paraLength"=w735, "pairIndex"=w736) -> ("is TDD11?"=w734:bool)  [unwired: 9 in]
                          n194 = case shown="假" w734 {
                            tunnel: w740 -> [w743 w745]
                            tunnel: [w742 w745] -> w739
                            tunnel: w738 -> [_ w744]
                            tunnel: ["TDD22" w744] -> w737
                            frame False {
                              n195 = Increment(x=w743) -> (x+1=w742:i32)
                            }
                            frame True {
                            }
                          }
                        }
                        frame "TDD22" {
                          n196 = local read "sparaLength"() -> (w748:dbl)
                          n197 = call "TDD11_22_seperate.vi"("paraLength"=w748, "pairIndex"=w747) -> ("is TDD11?"=w746:bool)  [unwired: 9 in]
                          n198 = case shown="假" w746 {
                            tunnel: w752 -> [w755 w757]
                            tunnel: [w754 w757] -> w751
                            tunnel: w750 -> [_ w756]
                            tunnel: ["TDD11" w756] -> w749
                            frame False {
                              n199 = Decrement(x=w755) -> (x-1=w754:i32)
                            }
                            frame True {
                            }
                          }
                        }
                      }
                      n200 = local read "Graph Size"() -> (w725:i32)
                      n201 = property class="Str"(reference=w722) -> (reference out=w720:refnum<vi>, "Value"=w721:string)  [unwired: 1 in, 1 out]
                      n202 = call "Graph Data Insert.vi"("Test Graph"=w731, "Item Name"=w704, "Graph Index"=w703, "Loop Index"=w705, "Limit Data"=w730, "Data"=w729, "Pair Loop"=w712, "Pair Name"=w726, "Graph Size"=w725) -> ()  [unwired: 11 in]
                      n203 = local read "proBar_ref"() -> (w709:refnum<vi>)
                      n204 = Search and Replace String(replace all?=TRUE ("替换全部？(F)"), input string=w723, search string="\r", replace string=w714) -> (result string=w718:string)  [unwired: 4 in, 3 out]
                      n205 = call "Summary Generating.vi"("Summary Method"=w727, "Status String"=w728, "String 2"=w723) -> ()  [unwired: 25 in]
                      n206 = Search and Replace String(replace all?=TRUE ("替换全部？(F)"), input string=w718, search string="\n", replace string=w714) -> (result string=w713:string)  [unwired: 4 in, 3 out]
                      n207 = property class="Slide (严格)"(reference=w709) -> ("Value"=w710:dbl)  [unwired: 1 in, 2 out]
                      n208 = Concatenate Strings(w721, w713, w714) -> (w719:string)
                      n209 = Add(x=w708, y=w710) -> (x+y=w711:dbl)
                      n210 = property class="Slide (严格)"(reference=w709, "Value"=w711) -> ()  [unwired: 1 in, 2 out]
                      n211 = property class="Str"(reference=w720, "Value"=w719) -> ()  [unwired: 1 in, 2 out]
                    }
                    frame True {
                      "ILD_15 graph index" <- w758
                    }
                  }
                }
                frame #3 {
                  n212 = Wait (ms)(milliseconds to wait=u32 200 ("等待时间（毫秒）")) -> ()  [unwired: 1 out]
                }
              }
              n213 = global read "全局.vi" "manual stop"() -> (w288:bool)
              n214 = Or(x=w289, y=w288) -> (x .or. y?=w287:bool)
            }
          }
          frame #3 {
            n215 = local read "sparaLength"() -> (w762:dbl)
            n216 = call "TDD11_22_seperate.vi"("paraLength"=w762, "pairIndex"=w761) -> ("is TDD11?"=w760:bool)  [unwired: 9 in]
            n217 = case shown="假" w760 {
              tunnel: w766 -> [w770 _]
              tunnel: [w769 w793] -> w765
              tunnel: [w768 w792] -> w763
              frame False {
                n218 = stacked-sequence {
                  seq-local: [w775 _] -> [_ w787]
                  seq-local: [w774 _] -> [_ w786]
                  tunnel: w770 -> [w779 _]
                  tunnel: [_ w788] -> w769
                  tunnel: [_ w785] -> w768
                  frame #0 {
                    n219 = local read "1d reslut"() -> (w773:bool[])
                    n220 = Search 1D Array(1D array=w779, element="TDD22" ("元素")) -> (index of element=w774:i32)  [unwired: 1 in]
                    n221 = Search 1D Array(1D array=w779, element="TDD11" ("元素")) -> (index of element=w775:i32)  [unwired: 1 in]
                    n222 = local read "Dataout"() -> (w778:dbl[][])
                    n223 = Index Array(array=w773, index=w774) -> (element=→"reslut_TDD22toTDD11 2":bool)
                    n224 = Index Array(array=w773, index=w775) -> (element=→"reslut_TDD11toTDD22":bool)
                    n225 = Index Array(array=w778, index (row)=w774) -> (element=→"TDD22toTDD11":dbl[])  [unwired: 1 in]
                    n226 = Index Array(array=w778, index (row)=w775) -> (element=→"TDD11toTDD22":dbl[])  [unwired: 1 in]
                  }
                  frame #1 {
                    n227 = local read "reslut_TDD22toTDD11 2"() -> (w783:bool)
                    n228 = local read "reslut_TDD11toTDD22"() -> (w782:bool)
                    n229 = local read "1d reslut"() -> (w784:bool[])
                    n230 = local read "TDD11toTDD22"() -> (w789:dbl[])
                    n231 = local read "TDD22toTDD11"() -> (w790:dbl[])
                    n232 = local read "Dataout"() -> (w791:dbl[][])
                    n233 = Replace Array Subset(array=w784, new element #1=w783, index #1=w787, new element #2=w782, index #2=w786) -> (w785:bool[])
                    n234 = Replace Array Subset(array=w791, new element #1=w790, index (row) #1=w787, new element #2=w789, index (row) #2=w786) -> (w788:dbl[][])  [unwired: 2 in]
                  }
                }
              }
              frame True {
                n235 = local read "Dataout"() -> (w793:dbl[][])
                n236 = local read "1d reslut"() -> (w792:bool[])
              }
            }
            "Dataout" <- w767
            "1d reslut" <- w764
          }
        }
        n237 = global read "全局.vi" "manual stop"() -> (w84:bool)
        n238 = Or(x=w85, y=w84) -> (x .or. y?=w83:bool)
      }
      "Result" <- w68
      "S4P_TXT_ Data" <- w61
      n239 = call "Data Retrim.vi"("Data in"=w52) -> ("Data Out"=→"Data Out":dbl[][][])  [unwired: 10 in]
    }
    frame #2 {
      n240 = local read "TXT Data Path"() -> (w808:path)
      n241 = local read "Frequency(Hz)"() -> (w803:dbl[])
      n242 = local read "Result"() -> (w811:bool[][])
      n243 = local read "Data Out"() -> (w809:dbl[][][])
      n244 = for {
        tunnel: w812 -> [w822] mode=indexing
        tunnel: w811 -> [w825]
        tunnel: w810 -> [w826]
        tunnel: [w820] -> w807 mode=indexing
        tunnel: w809 -> [w821] mode=indexing
        tunnel: w808 -> [w823]
        tunnel: [w819] -> w800 mode=indexing
        tunnel: [w818] -> w802 mode=indexing
        tunnel: w803 -> [w817]
        tunnel: w801 -> [w816]
        tunnel: [w815] -> w799 mode=indexing
        tunnel: w795 -> [w814]
        tunnel: w794 -> [w813]
        i -> [w824]
        n245 = stacked-sequence {
          seq-local: [w839 _ _] -> [_ w951 _]
          tunnel: w826 -> [w855 _ _]
          tunnel: w825 -> [w854 _ _]
          tunnel: w824 -> [w853 _ _]
          tunnel: w823 -> [w827 w950 _]
          tunnel: w822 -> [w835 w949 _]
          tunnel: w821 -> [w850 _ _]
          tunnel: [w830 _ _] -> w820
          tunnel: [w845 _ _] -> w819
          tunnel: [_ w956 _] -> w818
          tunnel: w817 -> [w844 _ _]
          tunnel: w816 -> [_ _ w958]
          tunnel: [w842 _ _] -> w815
          tunnel: w814 -> [w837 _ _]
          tunnel: w813 -> [w836 _ _]
          frame #0 {
            w856 = u16 0 items=["Normal Input", "Start", "Product Inf", "End"] ("Summary Method")
            n246 = call <vilib>:"Trim Whitespace.vi"("string"=w835) -> ("trimmed string"=w838:string)  [unwired: 1 in]
            n247 = case shown="\"ILD_15\"" w838 {
              selector: w838 -> [_ _ _ _ w899 _ _ _ _ _]
              tunnel: [w866 w876 w885 w892 w895 w914 w916 w929 w935 w946] -> w843
              tunnel: w850 -> [w868 w871 w882 w893 _ w915 w920 w933 w938 w945]
              tunnel: [w868 w870 w880 w893 w909 w915 w920 w933 w938 w944] -> w849
              tunnel: [w867 w877 w886 w889 w904 w913 w919 w932 w937 w941] -> w841
              tunnel: w844 -> [w866 w876 w885 w891 w895 _ _ _ _ _]
              tunnel: [TRUE TRUE TRUE TRUE w896 TRUE TRUE TRUE TRUE TRUE] -> w842
              tunnel: w837 -> [_ _ _ _ w902 _ _ _ _ _]
              tunnel: w836 -> [_ _ _ _ w898 _ _ _ _ _]
              tunnel: [TRUE TRUE TRUE TRUE w896 TRUE TRUE TRUE TRUE TRUE] -> w832
              tunnel: w827 -> [_ _ _ _ _ _ _ w924 _ _]
              frame "SDD21", Default {
                n248 = disable-structure shown="禁用" {
                  frame Disabled {
                    n249 = local write "SDD21 For ILD_15"(dbl[][] [] ("SDD21 For ILD_15")) -> ()
                  }
                  frame Enabled {
                  }
                }
                n250 = Array Size(array=w866) -> (size(s)=w867:i32)
                "大小" <- w867
              }
              frame "MDNEXT" {
                n251 = disable-structure shown="禁用" {
                  frame Disabled {
                    n252 = local write "SDD21 For ILD_15"(dbl[][] [] ("SDD21 For ILD_15")) -> ()
                  }
                  frame Enabled {
                  }
                }
                n253 = call-poly <userlib>:"Delete Elements from Array__ogtk.vi"("delete (rows or columns)"=enum16{"rows", "columns"}."rows", "indices"=i32[] [3, 7, 11, 15], "array"=w871) -> ("deleted elements"=w870:dbl[][])  [unwired: 7 in, 1 out]
                n254 = Array Size(array=w876) -> (size(s)=w877:i32)
              }
              frame "MDFEXT" {
                n255 = disable-structure shown="禁用" {
                  frame Disabled {
                    n256 = local write "SDD21 For ILD_15"(dbl[][] [] ("SDD21 For ILD_15")) -> ()
                  }
                  frame Enabled {
                  }
                }
                n257 = call-poly <userlib>:"Delete Elements from Array__ogtk.vi"("delete (rows or columns)"=enum16{"rows", "columns"}."columns", "indices"=i32[] [2, 5, 8, 11], "array"=w882) -> ("deleted elements"=w880:dbl[][])  [unwired: 7 in, 1 out]
                n258 = Array Size(array=w885) -> (size(s)=w886:i32)
              }
              frame "ILD" {
                n259 = disable-structure shown="禁用" {
                  frame Disabled {
                    n260 = local read "大小"() -> ()  [unwired: 1 out]
                  }
                  frame Enabled {
                  }
                }
                n261 = local read "Size"() -> (w889:i32)
                n262 = Array Subset(array=w891, length=w889) -> (w892:dbl[])  [unwired: 1 in]
              }
              frame "ILD_15" {
                (unwired) 0.15 ("ILD_spec")
                n263 = local read "2X Thru"() -> (w903:dbl[])
                n264 = local read "SDD21 For ILD_15"() -> (w901:dbl[][])
                n265 = local read "ILD_15 graph index"() -> (w900:i32)
                n266 = local read "大小"() -> (w908:i32)
                n267 = Subtract(x=w908, y=0) -> (x-y=w906:i32)
                n268 = Absolute Value(x=w906) -> (abs(x)=w904:i32)
                n269 = Array Subset(array=w901, length (col)=w904) -> (w905:dbl[][])  [unwired: 3 in]
                n270 = call "ILD_15%.vi"("Frequency(Hz)"=w895, "2x"=w903, "ILD data"=w905, "2x equalize"=w902) -> ("ILD_15% result"=w910:bool[], "ILD_15ChartData"=w894:T13, "ILD_15%"=w897:dbl[])  [unwired: 3 in]
                n271 = Build Array(w895, w897) -> (w909:dbl[][])
                n272 = And Array Elements(Boolean array=w910) -> (logical AND=w896:bool)
                n273 = call "ILD_15 graph.vi"("标题.文本"=w899, "Limit Data"=w894, "Graph Index"=w900, "Test Graph"=w898) -> ()  [unwired: 8 in]
              }
              frame "TDD11" {
                n274 = local read "Time Array"() -> (w914:dbl[])
                n275 = Array Size(array=w914) -> (size(s)=w913:i32)
              }
              frame "TCC11", "TCC22" {
                n276 = local read "Time Array 3"() -> (w916:dbl[])
                n277 = Array Size(array=w916) -> (size(s)=w919:i32)
              }
              frame "Delay" {
                n278 = local read "Time Array 4"() -> (w929:dbl[])
                n279 = local read "delay array"() -> (w928:dbl[])
                n280 = Concatenate Strings("delay_value" ("字符串"), ".txt" ("字符串")) -> (w926:string)
                n281 = Build Path(base path=w924, name or relative path=w926) -> (appended path=w922:path)
                n282 = Array Size(array=w929) -> (size(s)=w932:i32)
                n283 = call-poly <vilib>:"Write To Spreadsheet File.vi"("transpose? (no:F)"=TRUE, "format (%.3f)"="%.5f", "1D data"=w928, "file path (dialog if empty)"=w922) -> ()  [unwired: 4 in, 1 out]
              }
              frame "TDD22" {
                n284 = local read "Time Array 2"() -> (w935:dbl[])
                n285 = Array Size(array=w935) -> (size(s)=w937:i32)
              }
              frame "PSkew", "Pskew" {
                n286 = local read "Skew Time"() -> (w946:dbl[])
                n287 = local read "Skew result"() -> (w943:dbl[])
                n288 = Array Size(array=w946) -> (size(s)=w942:i32)
                n289 = call "Skew Data Process.vi"("Skew value"=w943, "Data Length"=w942, "Data In"=w945) -> ("Data out"=w944:dbl[][])  [unwired: 8 in]
                n290 = Increment(x=w942) -> (x+1=w941:i32)
              }
            }
            n291 = Index Array(array=w854, index (col)=w853) -> (element=w852:bool[])  [unwired: 1 in]
            n292 = And Array Elements(Boolean array=w852) -> (logical AND=w830:bool)
            n293 = Array Subset(array=w849, length (col)=w841) -> (w848:dbl[][])  [unwired: 3 in]
            n294 = Select(t="OK" ("字符串"), s=w830, f="NG" ("字符串")) -> (s? t:f=w845:string)
            n295 = Equal?(x=w835, y="ILD_15") -> (x = y?=w833:bool)
            n296 = Insert Into Array(array=w848, index (row)=0 ("索引 (行)"), new element=w843) -> (w840:dbl[][])  [unwired: 1 in]
            "ILD" <- w840
            n297 = Select(t=w832, s=w833, f=TRUE) -> (s? t:f=w829:bool)
            n298 = And(x=w830, y=w829) -> (x .and. y?=w828:bool)
            n299 = Select(t="Pass" ("字符串"), s=w828, f="Fail" ("字符串")) -> (s? t:f=w858:string)
            n300 = Concatenate Strings(w835, "_Total_Result:" ("字符串"), w858) -> (w857:string)
            n301 = call "Summary Generating.vi"("Summary Method"=w856, "Status String"=w855, "String 2"=w857) -> ()  [unwired: 25 in]
            n302 = case shown="\"SDD21\"" w835 {
              tunnel: w840 -> [w862 w863]
              tunnel: [w862 w863] -> w839
              frame "www", Default {
              }
              frame "SDD21" {
                "SDD21 For ILD_15" <- w863
              }
            }
          }
          frame #1 {
            n303 = call <vilib>:"Trim Whitespace.vi"("string"=w949) -> ("trimmed string"=w948:string)  [unwired: 1 in]
            n304 = Concatenate Strings(w948, ".txt" ("字符串")) -> (w953:string)
            n305 = Build Path(base path=w950, name or relative path=w953) -> (appended path=w955:path)
            n306 = call-poly <vilib>:"Write To Spreadsheet File.vi"("transpose? (no:F)"=TRUE, "format (%.3f)"="%.5f", "2D data"=w951, "file path (dialog if empty)"=w955) -> ()  [unwired: 4 in, 1 out]
            n307 = Array To Spreadsheet String(array=w951, 3:"%s" ("格式字符串")) -> (spreadsheet string=w956:string)  [unwired: 1 in]
          }
          frame #2 {
            n308 = case shown="\"E5071C\", 默认" w958 {
              frame "E5071C", Default {
              }
              frame "N5224A" {
              }
            }
          }
        }
      }
      "Testing Results" <- w807
      "Items Result" <- w800
      "ILD_15%" <- w799
      n309 = And Array Elements(Boolean array=w807) -> (logical AND=w797:bool)
      n310 = Array To Spreadsheet String(delimiter (Tab)="*" ("分隔符(Tab)"), array=w802, 3:"%s" ("格式字符串")) -> (spreadsheet string=→"String data":string)
      n311 = And Array Elements(Boolean array=w799) -> (logical AND=w798:bool)
      n312 = And(x=w797, y=w798) -> (x .and. y?=→"Total Reult":bool)
    }
    frame #3 {
      n313 = local read "TXT Data Path"() -> (w960:path)
      n314 = case shown="真" w959 {
        tunnel: w960 -> [_ w961]
        frame False {
        }
        frame True {
          n315 = property on="S4P Data Type" class="Enum (严格)"() -> ("RingText.Text"=w963:string)  [unwired: 2 in, 2 out]
          n316 = Concatenate Strings(w963, "_All_Txt_Data.txt" ("字符串")) -> (w969:string)
          n317 = Concatenate Strings(w963, "_All_S4P_Data.txt" ("字符串")) -> (w965:string)
          n318 = Build Path(base path=w961, name or relative path=w969) -> (appended path=w967:path)
          n319 = Build Path(base path=w961, name or relative path=w965) -> (appended path=w964:path)
          n320 = local read "S4P_TXT_ Data"() -> (w962:string[])
          n321 = local read "String data"() -> (w970:string)
          n322 = Write to Text File(file (use dialog)=w967, text=w970) -> ()  [unwired: 2 in, 3 out]
          n323 = call-poly <vilib>:"Write To Spreadsheet File.vi"("1D data"=w962, "file path (dialog if empty)"=w964) -> ()  [unwired: 6 in, 1 out]
        }
      }
    }
  }
